vi "Process.vi"(9 "process sync":refnum<notifier>, 11 "Main in":refnum<class "Main.lvclass">) -> ()   [LabVIEW 2019, in "Main.lvclass"]
doc: "Developed by Kevin Thompson\nkevin@thompsonengineering.net\n\nCopyright 2018\nThompson Engineering, LLC"
uses:
  Main.lvclass
  <vilib>/TELLC/SMQ/Add States to Queue using MultiLine String with vData.vi
  DataTypes/Process - AppData--cluster.ctl
  Common/DataTypes/TD Async CmdMsg EventData--cluster.ctl
  DataTypes/Public Events--cluster.ctl
  DataTypes/Dependency--cluster.ctl
  DataTypes/Settings--cluster.ctl
  Log_Engine/Log_Engine.lvclass
  DAQ_Engine/DAQ_Engine.lvclass
  Config/Config.lvclass
  Common/DataTypes/RawChannelData--cluster.ctl
  Common/DataTypes/RawDAQData--cluster.ctl
  Common/DataTypes/ChannelWaveforms--cluster.ctl
  Common/DataTypes/InverterWaveforms--cluster.ctl
  Common/DataTypes/InverterWaveforms--QRef.ctl
  Common/DataTypes/RawDAQDataQRef--cluster.ctl
  support/Data Algorithms/subvis/DataTypes/averaging variables.ctl
  support/Data Algorithms/subvis/DataTypes/ESR alarm variables.ctl
  support/Data Algorithms/subvis/DataTypes/Processing loop variables--cluster.ctl
  DataTypes/PrivateAsynEv_Main--enum.ctl
  Common/DataTypes/Measurement Config--cluster.ctl
  Common/DataTypes/DAQState--enum.ctl
  Common/DataTypes/Acquisition Mode--cluster.ctl
  support/Data Algorithms/subvis/DataTypes/Gain control.ctl
  Common/DataTypes/TDMSState--enum.ctl
  Common/DataTypes/LogState--enum.ctl
  Common/DataTypes/UpdateControlValue EvData--cluster.ctl
  support/Data Algorithms/subvis/DataTypes/ESR scaling--cluster.ctl
  DataTypes/DataProcessAuxData--cluster.ctl
  Common/DataTypes/DataProcAuxDat--Qref.ctl
  DataTypes/ProcessingState--enum.ctl
  DataTypes/ProcessingStateChg EvData--cluster.ctl
  DataTypes/InverterInfo--cluster.ctl
  DataTypes/ProcessInitParams--cluster.ctl
  DataTypes/StartProcInitParams--cluster.ctl
  Common/DataTypes/inverter offset range--cluster.ctl
  Common/DataTypes/inverter gain range--cluster.ctl
  Common/DataTypes/inverter info v2--cluster.ctl
  Common/DataTypes/Inverter database record v2--cluster.ctl
panel:
  in  "Data Rate 9775(S/s)":dbl=3.0 format="%#.6p"
  out "DAQ data":T1
  out "RawDaqDataQ size":i32
  in  "reset averaging":bool
  in  "Dummy Vrms":dbl=120.0
  in  "UseDummyVrms":bool
  in  "ESR scaling":T3[](array[typedef])
  in  "Data Rate 9215 (S/s)":dbl=1200000.0 format="%#.6p"
  in  "Signal scaling":T4[](array[typedef])
  in  "Exit":bool
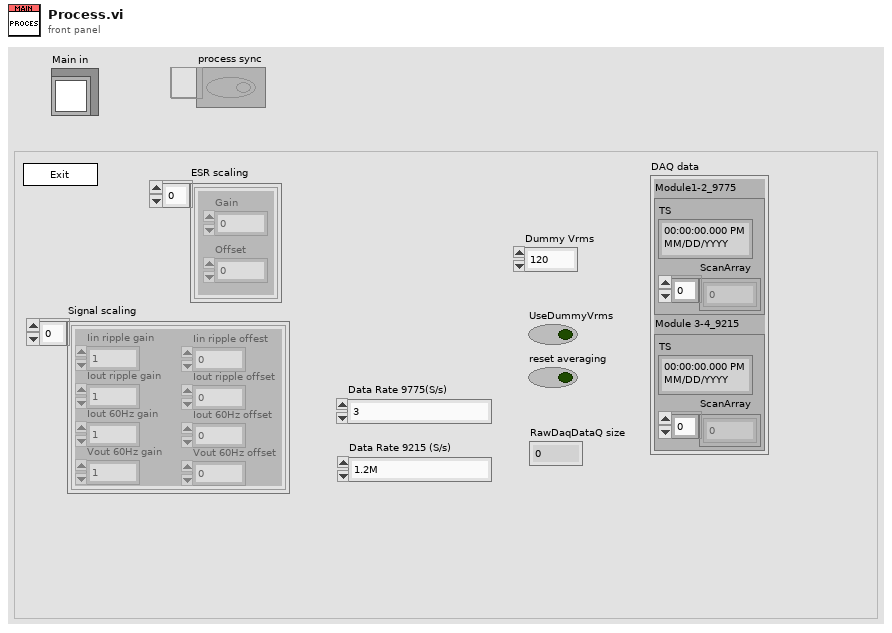
[diagram p1: front panel]
types:
  T1 = typedef "RawDAQData--cluster.ctl" = cluster{"Module1-2_9775":T2, "Module 3-4_9215":T2}
  T2 = typedef "RawChannelData--cluster.ctl" = cluster{"TS":timestamp, "ScanArray":dbl[]}
  T3 = typedef "Main.lvclass/ESR scaling--cluster.ctl" = cluster{"Gain":dbl, "Offset":dbl}
  T4 = typedef "Main.lvclass/Gain control.ctl" = cluster{"Iin ripple gain":dbl, "Iout ripple gain":dbl, "Iout 60Hz gain ":dbl, "Vout 60Hz gain ":dbl, "Iin ripple offest":dbl, "Iout ripple offset":dbl, "Iout 60Hz offset":dbl, "Vout 60Hz offset":dbl}
  T5 = typedef "Main.lvclass/ProcessingState--enum.ctl" = enum16{"Idle", "Starting", "Running", "Done", "Error"}
  T6 = typedef "Main.lvclass/Process - AppData--cluster.ctl" = cluster{"Core":cluster{"Current VI Reference":refnum<vi>, "Close Panel on Exit?":bool}, "Your Boolean data":bool, "Your string data":string, "SMQ":refnum<queue>, "Initialized?":bool, "Self Reference":refnum<class "Main.lvclass">, "Simulation?":bool, "process sync":refnum<notifier>, "vData":variant, "Settings":T7, "Dependency":T8, "Public Events":T9, "RawDaqDataQ":T10, "InverterWaveformsQ":T11, "Processing loop variables":T12, "Measurement config":T19, "Acquisition mode":T20, "DAQState":T21, "Signal scaling":T4, "PrivateAsync Ev":refnum<user-event>, "LogState":T22, "TDMSState":T23, "InvWfmsQ-DT":T11, "DPAuxDataQ":T24, "ProcessingState":T5, "InverterInfo":T25, "ProcLoopInterval":u32, "StoredESR Baseline":dbl[], "StoreESR BLine Flag":bool, "UseSavedESR BLine Flag":bool}
  T7 = typedef "Main.lvclass/Settings--cluster.ctl" = cluster{"Simulation":bool, "Signal scaling":T4[], "ESR scaling":T3[], "num readings to average":i32[], "ESR alarm threshhold (%)":i32[], "UseDummyVrms":bool, "Dummy Vrms":dbl, "Inverter Database File":path, "default Inverter (name)":string[], "Minimum Current Threshold ":dbl[], "Sensors Database File":path, "default Sensors (name)":string[]}
  T8 = typedef "Main.lvclass/Dependency--cluster.ctl" = cluster{"Config":refnum<class "Config.lvclass">, "DAQ":refnum<class "DAQ_Engine.lvclass">, "Log_Engine":refnum<class "Log_Engine.lvclass">}
  T9 = typedef "Main.lvclass/Public Events--cluster.ctl" = cluster{"Main.AsyncCmd Event":refnum<user-event>, "Main.AsyncMsg Event":refnum<user-event>, "stop process":refnum<user-event>, "UpdateControlValue Ev":refnum<user-event>, "ProcessingStateChg Ev":refnum<user-event>}
  T10 = typedef "RawDAQDataQRef--cluster.ctl" = refnum<queue>
  T11 = typedef "InverterWaveforms--QRef.ctl" = refnum<queue>
  T12 = typedef "Main.lvclass/Processing loop variables--cluster.ctl" = cluster{"DUT ESR avg":T13[], "DUT  PF avg":T13[], "DUT  Power avg ":T13[], "DUT processed data":cluster{"raw ESR":dbl, "Tcomp, avg ESR":dbl, "Vout RMS":dbl, "Iout RMS":dbl, "power factor":dbl, "power":dbl, "efficiency":dbl}[], "ESR alarm variables":T14[], "Status data":cluster{"Inv. 1 on?":bool, "Inv. 1 ESR over threshhold?":bool, "Minimum current":dbl}[], "CurrInverter":T15[], "miscellaneous":cluster{"Inverter 1 ID":string, "Inverter 2 ID":string, "Packet count":u32, "Calibration":dbl, "Calibration Gain":dbl, "Calibration Offset":dbl, "Calculated Total Power":dbl, "Seconds":dbl, "Last Tag Event":dbl, "Tag Event Time":dbl}[], "DUT INVERTER data":cluster{"Raw ESR sum":dbl, "scaled raw ESR sum":dbl, "scaled and averaged raw ESR sum":dbl, "Total power":dbl}[]}
  T13 = typedef "Main.lvclass/averaging variables.ctl" = cluster{"raw value buffer":dbl[], "buffer index":i32, "Avg value":dbl, "num to avg":i32}
  T14 = typedef "Main.lvclass/ESR alarm variables.ctl" = cluster{"Inv 1 baseline ESR":dbl, "Inv 1 over threshold?":bool, "Alarm on?":bool, "inv 1 esr chart range":dbl, "inv 1 esr saved baseline":dbl, "ESR alarm threshhold":dbl}
  T15 = typedef "Inverter database record v2--cluster.ctl" = cluster{"name":string, "last updated":timestamp, "type":string, "inverter Info":T16, "gain range":T17, "offset range":T18, "gain actual":dbl, "offset actual":dbl, "power level":dbl, "minimum current":dbl, "resistance single phase":dbl, "resistance 3 phase":dbl, "set flag":u16}
  T16 = typedef "inverter info v2--cluster.ctl" = cluster{"manufacturer":string, "model":string, "product":string, "serial":string, "power class":string, "year manf":string}
  T17 = typedef "inverter gain range--cluster.ctl" = cluster{"gain max":dbl, "gain min":dbl, "gain increment":dbl}
  T18 = typedef "inverter offset range--cluster.ctl" = cluster{"offset max":dbl, "offset min":dbl, "offset increment":dbl}
  T19 = typedef "Measurement Config--cluster.ctl" = cluster{"Data Rate 9775":dbl, "Data Rate 9215":dbl, "Samples RMS 9215":u32, "Samples RMS 9775":u32}
  T20 = typedef "Acquisition Mode--cluster.ctl" = enum16{"3phase", "Single"}
  T21 = typedef "DAQState--enum.ctl" = enum16{"Unknown", "Stopped", "Running", "Error"}
  T22 = typedef "LogState--enum.ctl" = enum16{"Unknown", "Stopped", "Running", "Error"}
  T23 = typedef "TDMSState--enum.ctl" = enum16{"Unknown", "Stopped", "Running", "Error"}
  T24 = typedef "DataProcAuxDat--Qref.ctl" = refnum<queue>
  T25 = typedef "InverterInfo--cluster.ctl" = cluster{"Inverter ID":string}
  T26 = typedef "Main.lvclass/ObjData--cluster.ctl" = cluster{"Settings":T7, "Public Events":T9, "Dependency":T8, "ReadData-placeholder":T27, "VISA-placeholder":refnum<visa-resource-name>, "InverterWaveformsQ":T11, "Application.TerminateProcess Event":refnum<user-event>, "RawDaqDataQ":T10, "MeasSettings":T19, "InverterDataAcqMode":T20, "DAQState Data":T28, "Private Events":T29, "InvWfmsQ-DT":T11, "DPAuxDataQ":T24, "ProcessingState":T5, "InverterInfo":T25, "CurrInverters":T15[], "InverterLUT Dict":T30, "ESR Chart Ref":refnum<vi>[], "StoreESR BLine Ref":refnum<vi>, "UseSavedESR BLine Ref":refnum<vi>, "CurrSensor":T31}
  T27 = typedef "Main.lvclass/Read Data--cluster.ctl" = cluster{"Data":dbl}
  T28 = typedef "DAQ_Engine.lvclass/DAQStateEvData--cluster.ctl" = cluster{"DAQState":T21, "vData":variant}
  T29 = typedef "Main.lvclass/Private Events--cluster.ctl" = cluster{"PrivateAsync Ev":refnum<user-event>}
  T30 = typedef "TD Dynamic CVT DVR--ref.ctl" = refnum<data-value>
  T31 = typedef "Sensor LUT--cluster.ctl" = cluster{"name":string, "last updated":timestamp, "manufacturer":string, "model":string, "Sensitivity index":dbl, "Sensor Ranges":T32}[]
  T32 = typedef "Sensor ranges--cluster.ctl" = cluster{"Max.VOut.RMS (V)":dbl, "Max.Out.Peak (V)":dbl, "Sensitivity (mV/A)":dbl, "Max.IOut.RMS(A)":dbl, "Min.IOut.RMS(A)":dbl}
  T33 = enum16{"Event Loop -", "Async Loop -", "DataProc Loop - "}
  T34 = typedef "Main.lvclass/PrivateAsynEv_Main--enum.ctl" = enum16{"PrivMain.UpdateMeasSettings", "PrivMain.UpdateAcqMode", "PrivMain.UpdateDAQState", "PrivMain.UpdateLogState", "PrivMain.UpdateTDMSState", "PrivMain.UpdateProcessingState", "PrivMain.Stop&Terminate", "PrivMain.CurrInverterUpdated", "PrivMain.UpdateStoreUseESRBaseline", "PrivMain.SetUnsetAlarm&ESRBLine", "PrivMain.ResetAveraging"}
  T35 = cluster{"VoltageDyn":dbl, "CurrentDyn":dbl, "MotorV SP":dbl}[]
  T36 = cluster{"Inv. 1 on?":bool, "Inv. 1 ESR over threshhold?":bool, "Minimum current":dbl}[]
  T37 = cluster{"Raw ESR sum":dbl, "scaled raw ESR sum":dbl, "scaled and averaged raw ESR sum":dbl, "Total power":dbl}[]
  T38 = typedef "InverterWaveforms--cluster.ctl" = T39[]
  T39 = typedef "ChannelWaveforms--cluster.ctl" = cluster{"Iin ripple ":waveform(dbl), "Iout ripple ":waveform(dbl), "Iout 60Hz":waveform(dbl), "Vout 60Hz":waveform(dbl)}
  T40 = typedef "DataProcessAuxData--cluster.ctl" = cluster{"Time Stamp":timestamp, "Raw ESR sum":dbl, "Inv 1 ON?":bool, "Average scaled ESR sum":dbl, "Inv 1 over threshold?":bool, "Inv 1 ESR":cluster{"ESR Baseline":dbl, "Alarm threshhold (%)":dbl, "Avg value":dbl}, "Max ESR":dbl}
  T41 = typedef "TD MeasData--cluster.ctl" = cluster{"Timestamp":timestamp, "ESR_Ohm":dbl[], "DUT data":T42[], "DUT INVERTER data":cluster{"Raw ESR sum":dbl, "scaled raw ESR sum":dbl, "scaled and averaged raw ESR sum":dbl, "Total power":dbl}[]}
  T42 = typedef "InverterPhaseData--cluster.ctl" = cluster{"RawESR_Ohm":dbl, "TcompAvgESR_Ohm":dbl, "VoutRMS_V":dbl, "IoutRMS_A":dbl, "PF":dbl, "AvgPF":dbl, "Power_W":dbl, "AvgPower_W":dbl, "efficiency":dbl}
  T43 = enum32{"invalid app kind", "Development System", "Run Time System", "Student Edition", "Embedded LabVIEW", "Evaluation", "Custom"}
  T44 = enum32{"Invalid", "Standard", "Closed", "Hidden", "Minimized", "Maximized"}
  T45 = cluster{"Inv. 1 on?":bool, "Inv. 1 ESR over threshhold?":bool, "Minimum current":dbl}
  T46 = cluster{"Inverter 1 ID":string, "Inverter 2 ID":string, "Packet count":u32, "Calibration":dbl, "Calibration Gain":dbl, "Calibration Offset":dbl, "Calculated Total Power":dbl, "Seconds":dbl, "Last Tag Event":dbl, "Tag Event Time":dbl}
  T47 = typedef "Main.lvclass/AsynCmd_Main--enum.ctl" = enum16{"Main.StartProcessing", "Main.StopProcessing", "Main.RefreshInverterList"}
  T48 = typedef "Main.lvclass/StartProcInitParams--cluster.ctl" = cluster{"InverterInfo":T25[], "ProcessInitParams":T49[]}
  T49 = typedef "Main.lvclass/ProcessInitParams--cluster.ctl" = cluster{"MinCurrThreshold":dbl, "NumPF RdsToAvg":i32, "ESR alarm threshhold (%)":dbl, "# readings to average":i32}
  T50 = typedef "Main.lvclass/AsynMsg_Main--enum.ctl" = enum16{"Main.CurrInverterUpdated"}
  T51 = typedef "DAQ_Engine.lvclass/DAQMeasSettingsEvData--cluster.ctl" = cluster{"Measurement config":T19, "vData":variant}
  T52 = typedef "Log_Engine.lvclass/LogStateEvData--cluster.ctl" = cluster{"LogState":T22, "vData":variant}
  T53 = typedef "Log_Engine.lvclass/TDMSStateEvData--cluster.ctl" = cluster{"TDMSState":T23, "vData":variant}
  T54 = typedef "DAQ_Engine.lvclass/Public Events--cluster.ctl" = cluster{"DAQ_Engine.AsyncCmd Event":refnum<user-event>, "DAQ_Engine.AsyncMsg Event":refnum<user-event>, "stop process":refnum<user-event>, "DAQ_Engine.DAQStateChg Ev":refnum<user-event>, "DAQ_Engine.MeasSettingsChg Ev":refnum<user-event>, "DAQ_Engine.AcqModeChg Ev":refnum<user-event>}
  T55 = typedef "Log_Engine.lvclass/Public Events--cluster.ctl" = cluster{"Log_Engine.AsyncCmd Event":refnum<user-event>, "Log_Engine.AsyncMsg Event":refnum<user-event>, "stop process":refnum<user-event>, "Log_Engine.LogStateChg Ev":refnum<user-event>, "Log_Engine.TDMSStateChg Ev":refnum<user-event>}
  T56 = cluster{"Current VI Reference":refnum<vi>, "Close Panel on Exit?":bool}
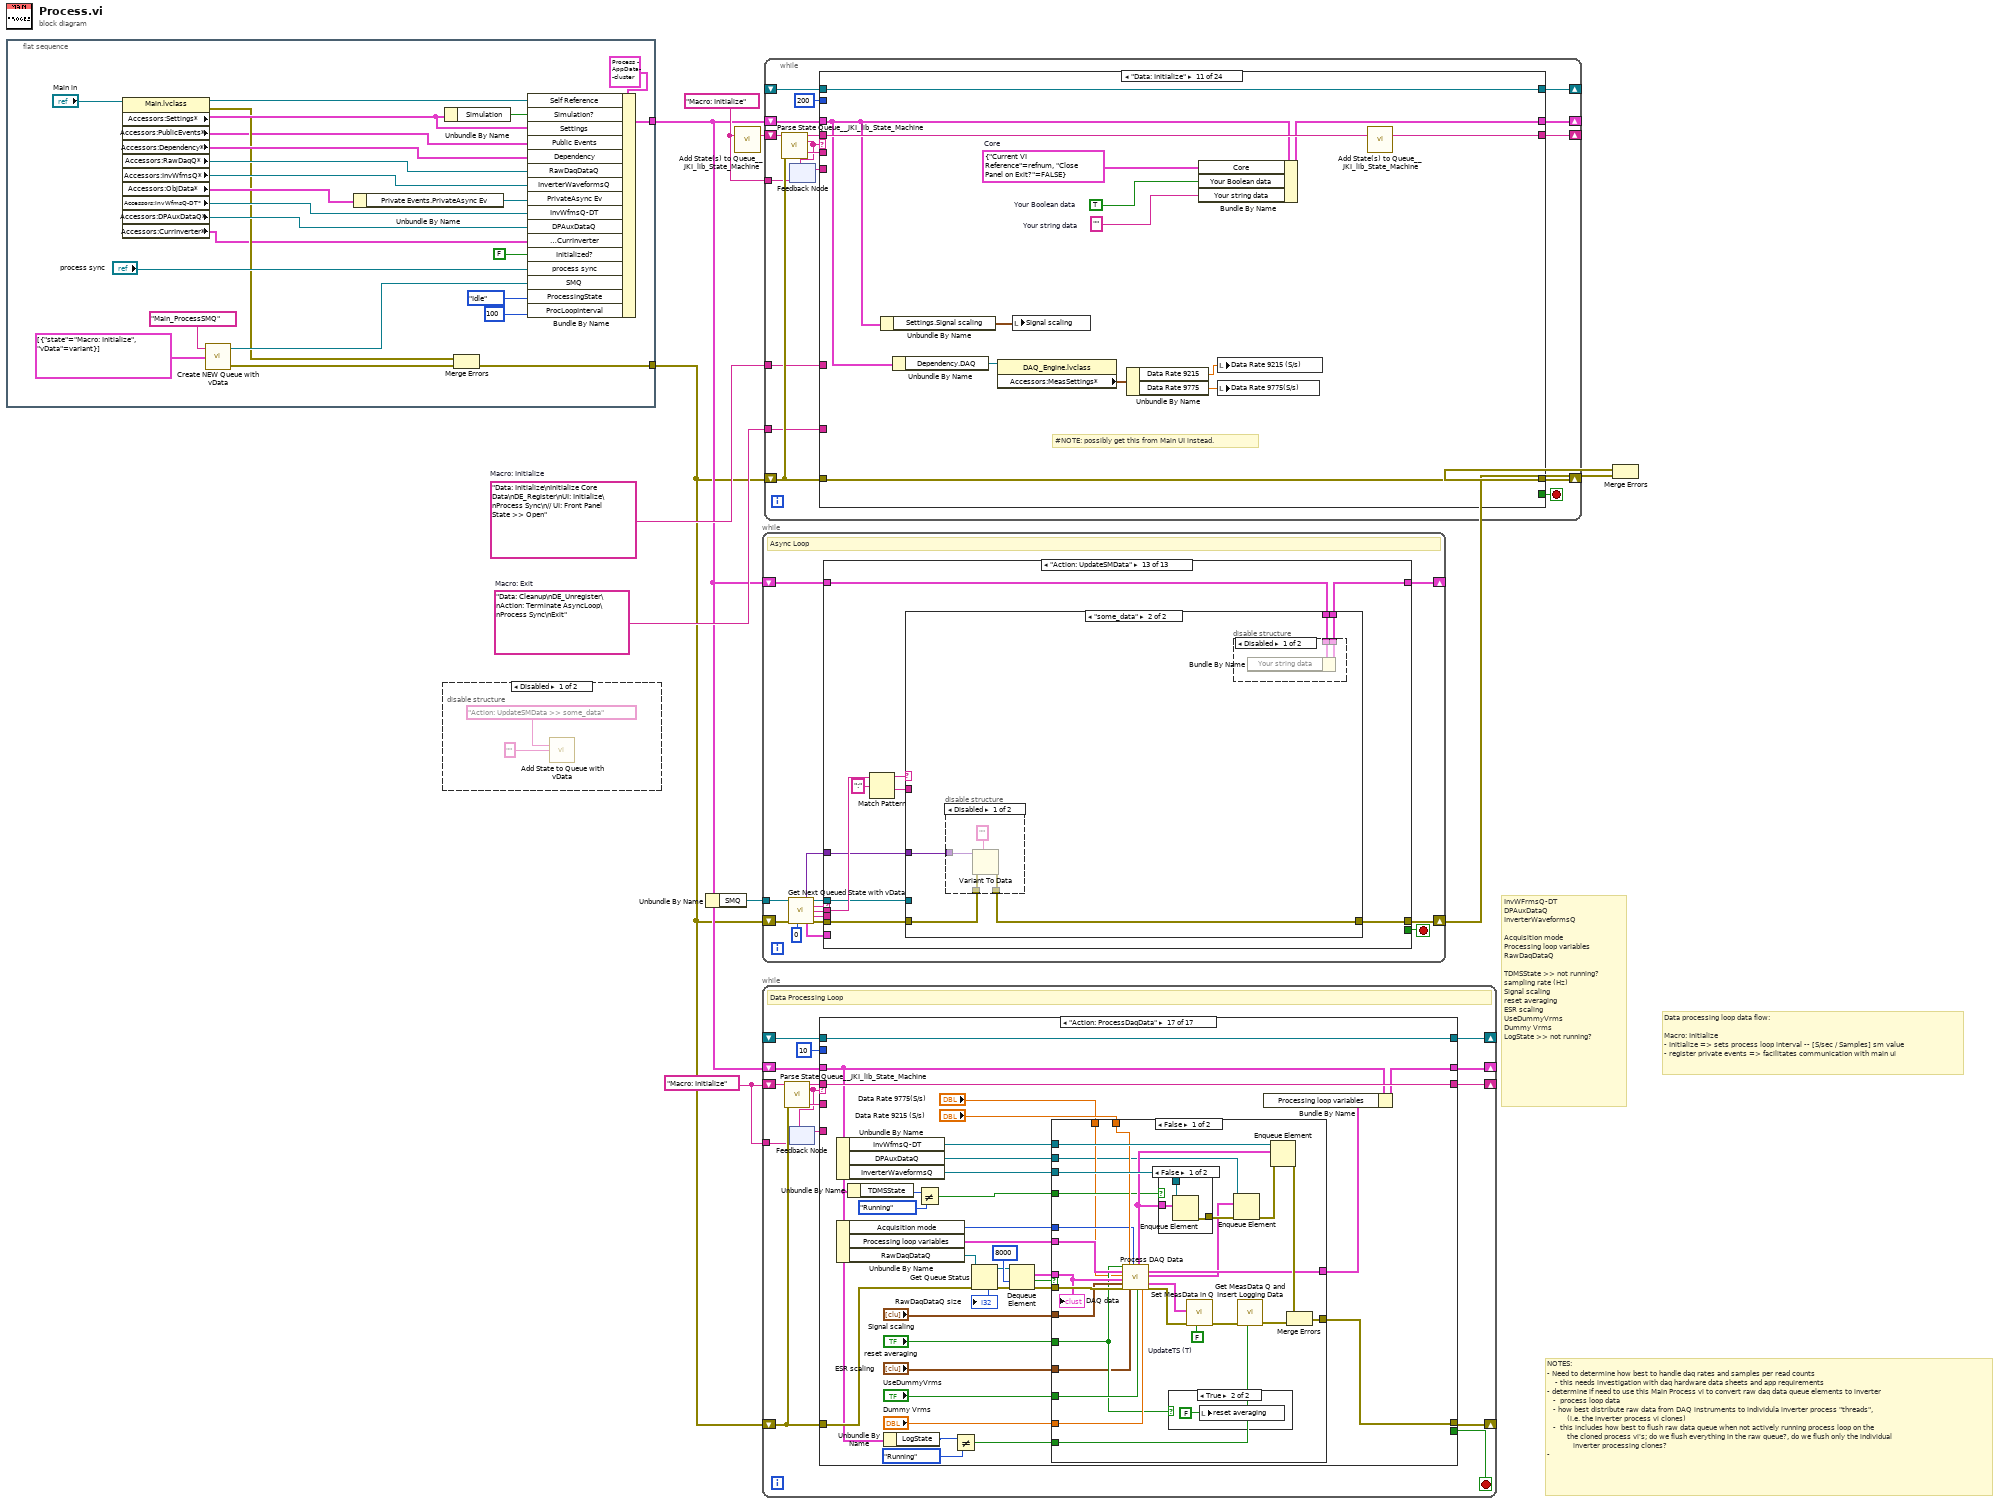
[diagram p0: block diagram]
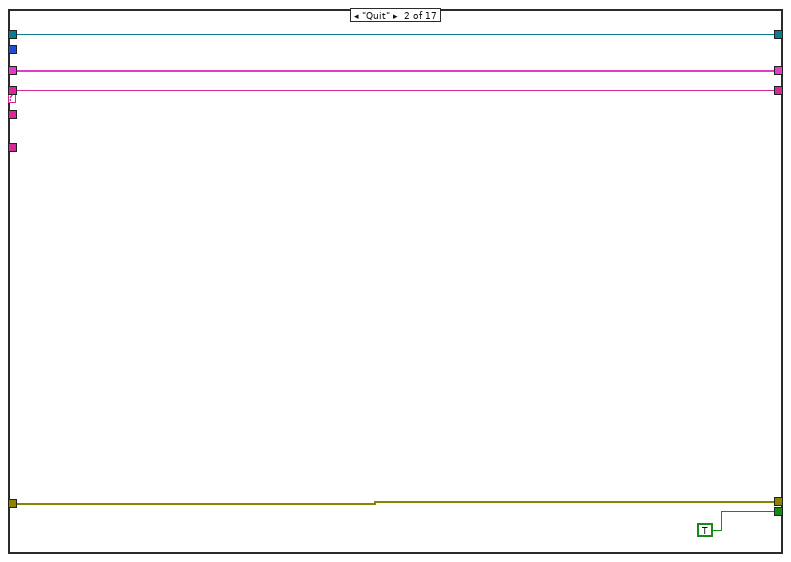
[diagram p3: hidden frame]
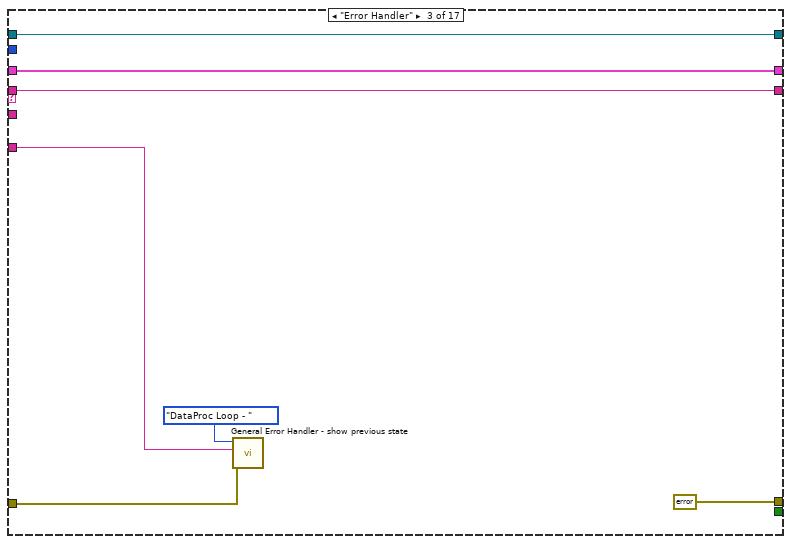
[diagram p4: hidden frame]
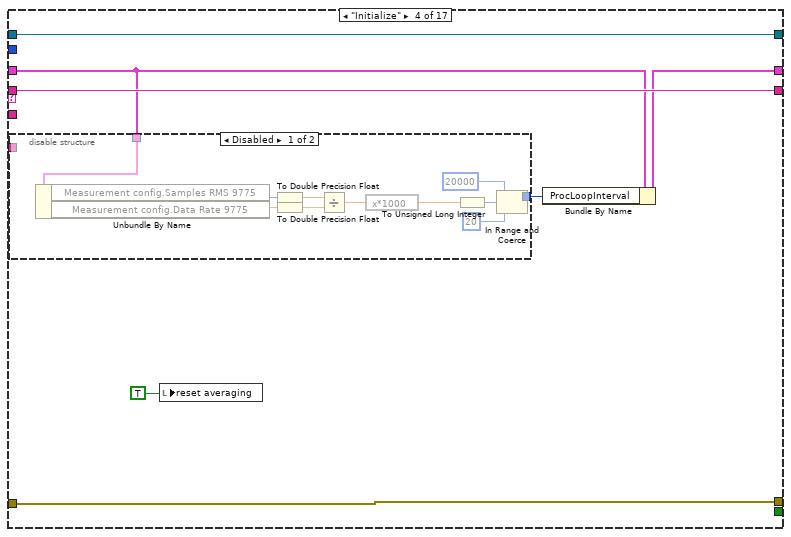
[diagram p5: hidden frame]
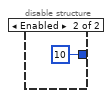
[diagram p6: hidden frame]
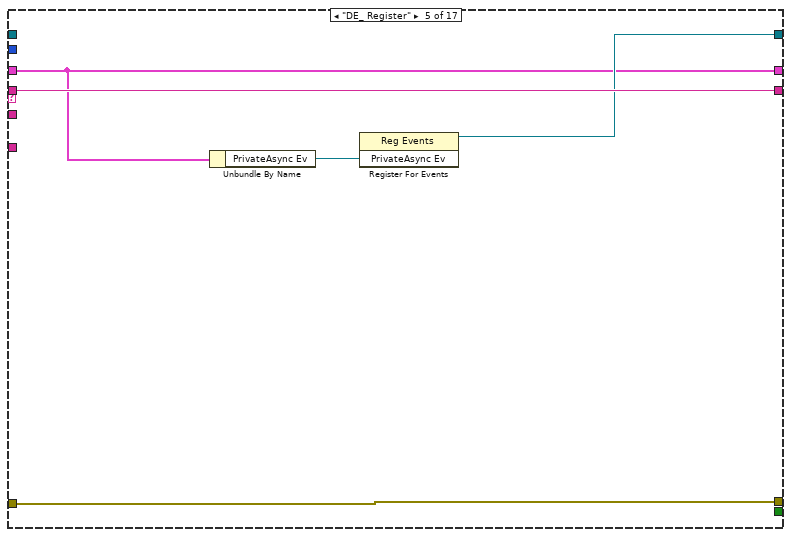
[diagram p7: hidden frame]
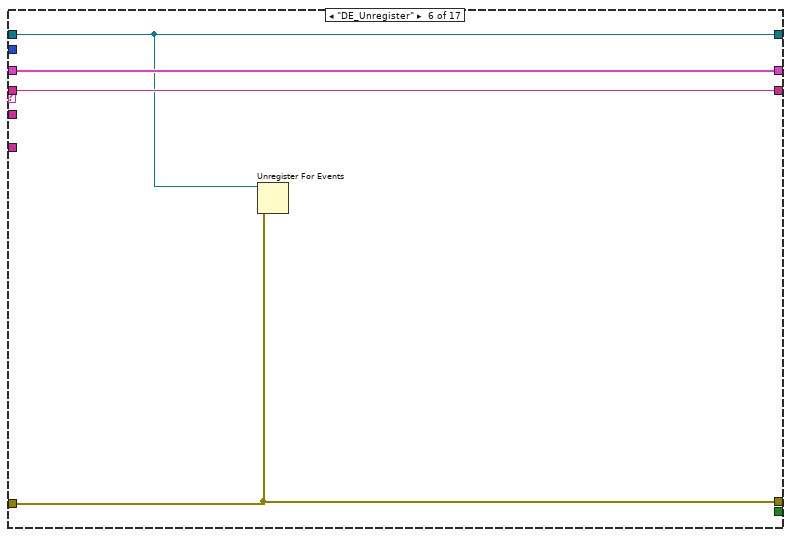
[diagram p8: hidden frame]
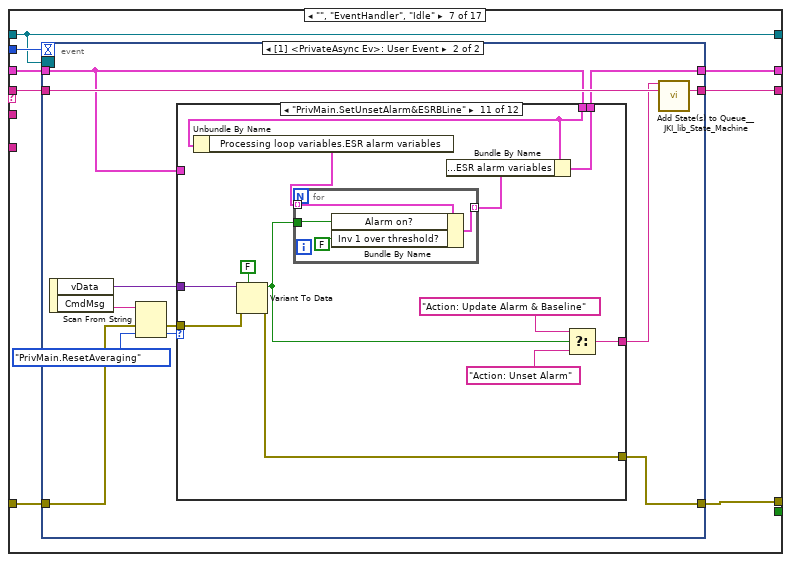
[diagram p9: hidden frame]
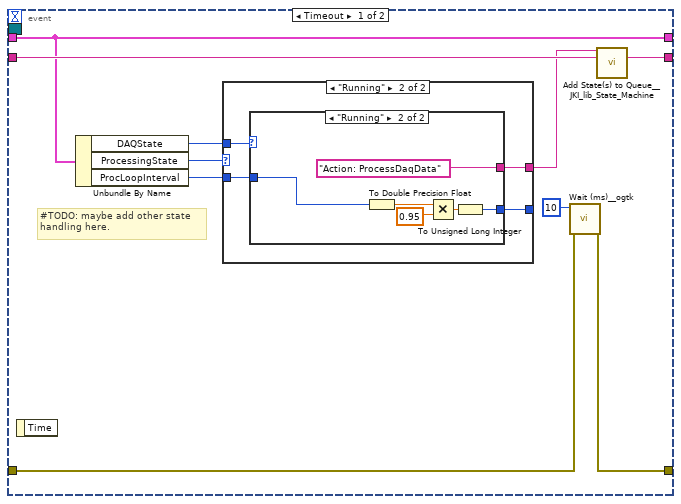
[diagram p10: hidden frame]
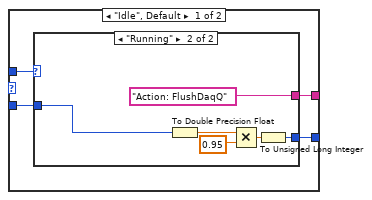
[diagram p11: hidden frame]
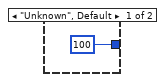
[diagram p12: hidden frame]
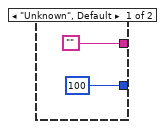
[diagram p13: hidden frame]
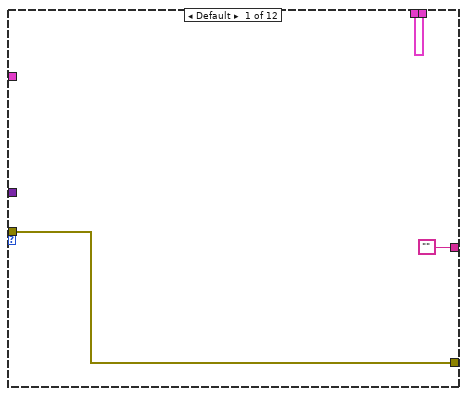
[diagram p14: hidden frame]
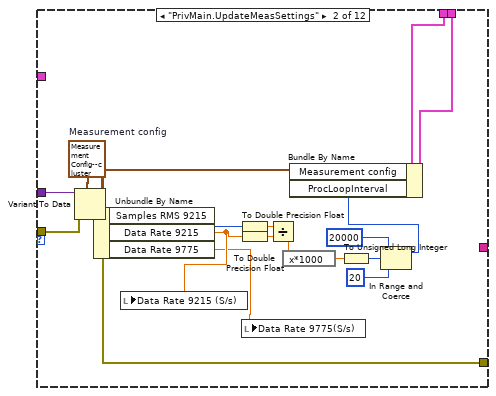
[diagram p15: hidden frame]
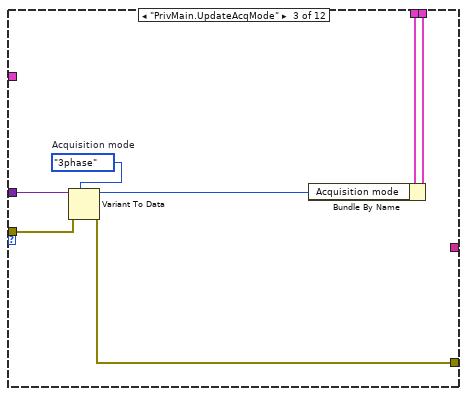
[diagram p16: hidden frame]
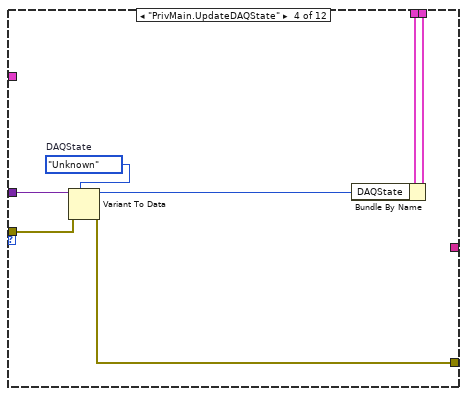
[diagram p17: hidden frame]
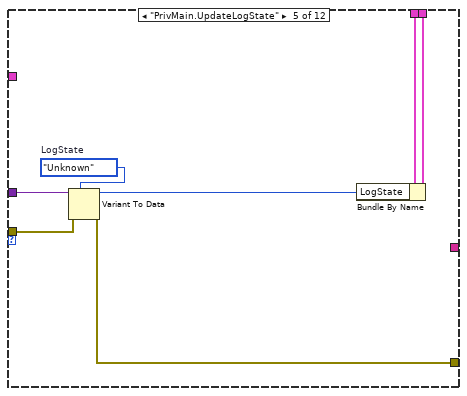
[diagram p18: hidden frame]
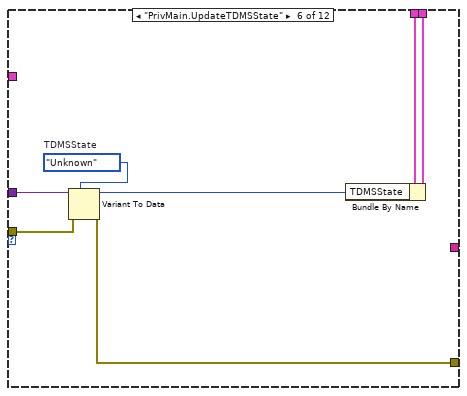
[diagram p19: hidden frame]
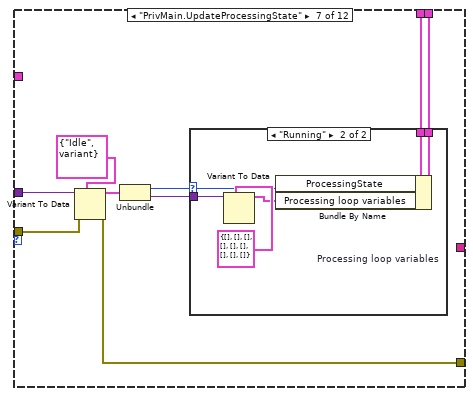
[diagram p20: hidden frame]
diagram:
  w1 = "Macro: Initialize"
  w8 = "Data: Cleanup\nDE_Unregister\nAction: Terminate AsyncLoop\nProcess Sync\nExit"  # Macro: Exit
  w9 = "Data: Initialize\nInitialize Core Data\nDE_Register\nUI: Initialize\nProcess Sync\n// UI: Front Panel State >> Open"  # Macro: Initialize
  w4 = "Macro: Initialize"
  # "NOTES:\n- Need to determine how best to handle daq rates and samples per read counts\n    - this needs investigation with daq hardware data sheets and app requirements\n- determine if need to use this Main Process vi to convert raw daq data queue elements to inverter\n   -  process loop data\n   - how best distribute raw data from DAQ instruments to individula inverter process \"threads\",\n          (i.e. the inverter process vi clones)\n   -  this includes how best to flush raw data queue when not actively running process loop on the\n          the cloned process vi's; do we flush everything in the raw queue?, do we flush only the individual\n             inverter processing clones?\n-"
  # "Data processing loop data flow:\n\nMacro: Initialize\n- Initialize => sets process loop interval -- [S/sec / Samples] sm value\n- register private events => facilitates communication with main ui"
  # "InvWFrmsQ-DT\nDPAuxDataQ\nInverterWaveformsQ\n\nAcquisition mode\nProcessing loop variables\nRawDaqDataQ\n\nTDMSState >> not running?\nsampling rate (Hz)\nSignal scaling\nreset averaging\nESR scaling\nUseDummyVrms\nDummy Vrms\nLogState >> not running?"
  n1 = flat-sequence {
    tunnel: [w35] -> w3
    tunnel: [w16] -> w2
    frame #0 {
      n2 = property class="Main.lvclass"(reference="Main in") -> (reference out=w14:refnum<class "Main.lvclass">, error out=w15:errorcluster, "Accessors:Settings*"=w26:T7, "Accessors:PublicEvents*"=w13:T9, "Accessors:Dependency*"=w28:T8, "Accessors:RawDaqQ*"=w24:T10, "Accessors:InvWfmsQ*"=w23:T11, "Accessors:ObjData*"=w22:T26, "Accessors:InvWfmsQ-DT*"=w20:T11, "Accessors:DPAuxDataQ*"=w19:T24, "Accessors:CurrInverter*"=w11:T15[])  [unwired: 1 in]
      n3 = call <vilib>:"Create NEW Queue with vData.vi"("Initial States"=cluster{"state":string, "vData":variant}[] [{"state"="Macro: Initialize", "vData"=variant}], "Name (SMQ)"="Main_ProcessSMQ") -> ("error out"=w32:errorcluster, "queue out"=w34:refnum<queue>)  [unwired: 2 in]
      n4 = Unbundle By Name(w22) -> ("Private Events.PrivateAsync Ev"=w21:refnum<user-event>)
      n5 = Unbundle By Name(w26) -> ("Simulation"=w27:bool)
      n6 = Merge Errors(w15, w32) -> (w16:errorcluster)
      n7 = Bundle By Name(cluster=T6 {"Core"={"Current VI Reference"=refnum, "Close Panel on Exit?"=FALSE}, "Your Boolean data"=FALSE, "Your string data"="", "SMQ"=refnum, "Initialized?"=FALSE, "Self Reference"=refnum, "Simulation?"=FALSE, "process sync"=refnum, "vData"=variant, "Settings"={"Simulation"=FALSE, "Signal scaling"=[], "ESR scaling"=[], "num readings to average"=[], "ESR alarm threshhold (%)"=[], "UseDummyVrms"=FALSE, "Dummy Vrms"=0.0, "Inverter Database File"=path "", "default Inverter (name)"=[], "Minimum Current Threshold "=[], "Sensors Database File"=path "", "default Sensors (name)"=[]}, "Dependency"={"Config"=refnum, "DAQ"=refnum, "Log_Engine"=refnum}, "Public Events"={"Main.AsyncCmd Event"=refnum, "Main.AsyncMsg Event"=refnum, "stop process"=refnum, "UpdateControlValue Ev"=refnum, "ProcessingStateChg Ev"=refnum}, "RawDaqDataQ"=refnum, "InverterWaveformsQ"=refnum, "Processing loop variables"={"DUT ESR avg"=[], "DUT  PF avg"=[], "DUT  Power avg "=[], "DUT processed data"=[], "ESR alarm variables"=[], "Status data"=[], "CurrInverter"=[], "miscellaneous"=[], "DUT INVERTER data"=[]}, "Measurement config"={"Data Rate 9775"=3.0, "Data Rate 9215"=1200000.0, "Samples RMS 9215"=480000, "Samples RMS 9775"=3}, "Acquisition mode"=enum."3phase", "DAQState"=enum."Unknown", "Signal scaling"={"Iin ripple gain"=13.333, "Iout ripple gain"=13.333, "Iout 60Hz gain "=14.286, "Vout 60Hz gain "=20.0, "Iin ripple offest"=0.0, "Iout ripple offset"=0.0, "Iout 60Hz offset"=0.0, "Vout 60Hz offset"=0.0}, "PrivateAsync Ev"=refnum, "LogState"=enum."Unknown", "TDMSState"=enum."Unknown", "InvWfmsQ-DT"=refnum, "DPAuxDataQ"=refnum, "ProcessingState"=enum."Idle", "InverterInfo"={"Inverter ID"=""}, "ProcLoopInterval"=0, "StoredESR Baseline"=[], "StoreESR BLine Flag"=FALSE, "UseSavedESR BLine Flag"=FALSE} ("SM2 AppData"), "Self Reference"=w14, "Simulation?"=w27, "Settings"=w26, "Public Events"=w13, "Dependency"=w28, "RawDaqDataQ"=w24, "InverterWaveformsQ"=w23, "PrivateAsync Ev"=w21, "InvWfmsQ-DT"=w20, "DPAuxDataQ"=w19, "Processing loop variables.CurrInverter"=w11, "Initialized?"=FALSE, "process sync"="process sync", "SMQ"=w34, "ProcessingState"=ProcessingState--enum."Idle", "ProcLoopInterval"=u32 100) -> (w35:T6)
    }
  }
  n8 = disable-structure shown="Disabled" {
    frame Disabled {
      n9 = call <vilib>:"Add State to Queue with vData.vi"("state in"="Action: UpdateSMData >> some_data", "vData (\"\")"="") -> ()  [unwired: 10 in, 4 out]
    }
    frame Enabled {
    }
  }
  n10 = Unbundle By Name(w3) -> ("SMQ"=w7:refnum<queue>)
  n11 = call <vilib>:"Add State(s) to Queue__JKI_lib_State_Machine.vi"("State(s) in (\"\")"=w4) -> ("States Out"=w10:string)  [unwired: 14 in]
  n12 = while {
    shift-right: [w48] -> w5
    shift-left: w2 -> [w50]
    tunnel: w7 -> [w46]
    shift-right: [w44] -> _
    shift-left: w3 -> [w45]
    stop <- w39 stop-if-true
    # "Async Loop"
    n13 = call <vilib>:"Get Next Queued State with vData.vi"("queue in"=w46, "error in (no error)"=w50, "timeout (100)"=0) -> ("vData out"=w43:variant, "queue out"=w47:refnum<queue>, "Next State"=w51:string, "queued msg"=w41:string, "Prev State"=w40:string, "RemainingElements"=w38:cluster{"state":string, "vData":variant}[], "error out"=w49:errorcluster)  [unwired: 6 in]
    n14 = case shown="\"Action: UpdateSMData\"" w51 {
      tunnel: w47 -> [_ _ _ _ w70 w80 _ w96 w101 _ _ _ w138]
      tunnel: w41 -> [_ _ _ _ _ _ _ _ _ _ _ w127 w140]
      selector: w51 -> [w52 _ _ _ _ _ _ _ _ _ _ _ _]
      tunnel: w49 -> [w54 w62 w64 w69 w76 w78 w92 w95 w100 w104 w106 w126 w135]
      tunnel: [w53 w62 errorcluster {"status"=FALSE, "code"=0, "source"=""} ("error constant") w69 w76 w77 w92 w94 w99 w104 w106 w129 w134] -> w48
      tunnel: w45 -> [w60 w61 w67 w68 w75 w79 w91 w97 w102 w103 w107 w132 w137]
      tunnel: [w60 w61 w67 w68 w75 w79 w91 w97 w102 w103 w107 w132 w136] -> w44
      tunnel: w43 -> [_ _ _ _ _ _ _ _ _ _ _ _ w139]
      tunnel: w40 -> [_ _ w63 _ _ _ _ _ _ _ _ _ _]
      tunnel: [_ _ _ _ TRUE _ _ _ _ _ _ _ _] -> w39
      tunnel: w38 -> [_ _ _ _ _ _ _ _ _ _ _ _ _]
      frame Default {
        w56 = 42 items=["No error", "Argument error", "Memory is full", "Out of zone", "End of file", "File already open", "Generic file I/O error", "File not found", "File permission error", "Disk is full", "Duplicate path", "Too many files open", "System feature not enabled", "Resource file not found", "Cannot add resource", "Resource not found", "Image not found", "Image memory error", "Pen does not exist", "Config type invalid", "Config token not found", "Config parse error", "Config memory error", "Bad external code format", "Bad external code offset", "External code not present", "Null window", "Destroy window error", "Null menu", "Print aborted", "Bad print record", "Print driver error", "Windows error during printing", "Memory error during printing", "Print dialog error", "Generic print error", "Invalid device refnum", "Device not found", "Device parameter error", "Device unit error", "Cannot open device", "Device call aborted", "Generic error", "Cancelled by user", "Object ID too low", "Object ID too high", "Object not in heap", "Unknown heap", "Unknown object (invalid DefProc)", "Unknown object (DefProc not in table)", "Message out of range", "Invalid (null) method", "Unknown message", "Manager call not supported", "Bad address", "Network operation in progress", "Network operation timed out", "Connection is busy", "Network attribute not supported", "Network error", "Address in use", "System out of memory", "Connection aborted", "Connection refused", "Not connected", "Already connected", "Connection closed", "Initialization error (interapplication manager)", "Bad occurrence", "Wait on unbound occurrence handler", "Occurrence queue overflow", "Datalog type conflict", "Unused", "Unrecognized type (interapplication manager)", "Memory corrupt", "Failed to make temporary DLL", "Old CIN version", "Drag socket not found", "Failed to load drop-object", "Failed to register OLE object", "Failed to release OLE object", "Format specifier type mismatch", "Unknown format specifier", "Too few format specifiers", "Too many format specifiers", "Scan failed", "Newer CIN version", "Error converting to variant", "Runtime menu error", "Password tampered", "Variant attribute not found", "Incompatible variant data type", "Event data is not available", "Event Store is not present", "Occurrence is not found", "Event Queue is not created", "Event info is not available", "Refnum passed is NULL", "Error retrieving Class GUID", "Error retrieving CoClass GUID", "Error retrieving TypeLib GUID.", "Bad built application magic bytes.", "Specific driver is different from the specific driver associated with the Logical Name.", "There is no session opened to the class driver.", "Max Error", "MAX - Error with config objects", "MAX - Error loading configuration", "MAX - Group not supported"]
        n15 = Format Into String(format string="Software Exception: Unhandled State \"%s\"." ("message"), error in=w54, w52) -> (resulting string=w57:string, error out=w58:errorcluster)  [unwired: 1 in]
        n16 = call <vilib>:"Error Cluster From Error Code.vi"("show call chain? (False)"=TRUE, "error in (no error)"=w58, "error message (\"\")"=w57, "error code (0)"=w56) -> ("error out"=w53:errorcluster)  [unwired: 5 in]
      }
      frame "Initialize" {
      }
      frame "Error Handler" {
        n17 = call "General Error Handler - show previous state.vi"("error in (no error)"=w64, "Previous State"=w63, "Loop Select"=enum16{"Event Loop -", "Async Loop -"}."Async Loop -") -> ()  [unwired: 7 in, 2 out]
      }
      frame "CleanUp" {
      }
      frame "Exit" {
        n18 = Flush Queue(queue=w70) -> (queue out=w73:refnum<queue>, error out=w72:errorcluster)  [unwired: 1 in, 1 out]
        n19 = Release Queue(queue=w73, force destroy? (F)=TRUE, error in (no error)=w72) -> ()  [unwired: 3 out]
      }
      frame "", "Idle" {
        # "#NOTE: This Async Loop NOT USED in this app.\nNeeded faster response; see bottom loop.\nCode remains here for reference and re-use if needed."
        # "#TODO: add condition"
        n20 = Unbundle By Name(w79) -> ()  [unwired: 1 out]
        n21 = case shown="False" FALSE {
          tunnel: w80 -> [_ w90]
          tunnel: w78 -> [w83 w87]
          tunnel: [w82 w85] -> w77
          frame False {
            n22 = call <userlib>:"Wait (ms)__ogtk.vi"("error in (no error)"=w83, "milliseconds to wait"=u32 200) -> ("error out"=w82:errorcluster)  [unwired: 8 in, 1 out]
          }
          frame True {
            n23 = call <userlib>:"Wait (ms)__ogtk.vi"("error in (no error)"=w87, "milliseconds to wait"=u32 50) -> ("error out"=w88:errorcluster)  [unwired: 8 in, 1 out]
            n24 = call-poly <vilib>:"Polymorphic - Add States(s) To Queue.vi"("queue in"=w90, "state in"="Action: ReadRawDaqQueue", "error in"=w88) -> ("error out"=w85:errorcluster)  [unwired: 9 in, 3 out]
          }
        }
      }
      frame "------ Macro ------" {
      }
      frame "Macro: Initialize" {
        n25 = call-poly <vilib>:"Polymorphic - Add States(s) To Queue.vi"("queue in"=w96, "states in"="Initialize\n/* some state\n/* another state\nIdle", "error in"=w95) -> ("error out"=w94:errorcluster)  [unwired: 10 in, 2 out]
      }
      frame "Macro: Exit" {
        n26 = call-poly <vilib>:"Polymorphic - Add States(s) To Queue.vi"("queue in"=w101, "states in"="/* some state\n/* another state\nCleanUp\nExit", "error in"=w100) -> ("error out"=w99:errorcluster)  [unwired: 10 in, 2 out]
      }
      frame "------ Action ------" {
      }
      frame "Action: ReadRawDaqQueue" {
        n27 = Unbundle By Name(w107) -> ("RawDaqDataQ"=w105:T10)
        n28 = disable-structure shown="Disabled" {
          disable-tunnel: w105 -> [_ w108 w119]
          frame Enabled {
          }
          frame Disabled {
            n29 = Get Queue Status(queue=w108) -> (queue out=w110:T10, error out=w109:errorcluster, # elements in queue=w111:i32)  [unwired: 2 in, 5 out]
            n30 = case shown="1, Default" w111 {
              selector: w111 -> [_ w114]
              tunnel: w110 -> [_ w113]
              tunnel: w109 -> [_ w112]
              frame 0 {
              }
              frame 1, Default {
                n31 = for {
                  N: w114 -> [_]
                  tunnel: w113 -> [w118]
                  shift-right: [w116] -> _
                  shift-left: w112 -> [w117]
                  tunnel: [w115] -> _ mode=indexing
                  n32 = Dequeue Element(queue=w118, error in (no error)=w117) -> (element=w115:T1, error out=w116:errorcluster)  [unwired: 1 in, 2 out]
                }
              }
            }
          }
          frame Disabled {
            n33 = while {
              tunnel: w119 -> [w124]
              stop <- w123 stop-if-true
              n34 = Dequeue Element(queue=w124, timeout in ms (-1)=5) -> (timed out?=w122:bool, error out=w121:errorcluster)  [unwired: 1 in, 2 out]
              n35 = Compound Arithmetic op=OR(w122, w121) -> (w123:bool)
            }
          }
        }
      }
      frame "Action: Wait" {
        n36 = Scan From String(format string="%d", input string=w127, error in=w126, default 1=u32 0) -> (error out=w125:errorcluster, output 1=w131:u32)  [unwired: 1 in, 2 out]
        n37 = call <userlib>:"Wait (ms)__ogtk.vi"("error in (no error)"=w125, "milliseconds to wait"=w131) -> ("error out"=w129:errorcluster)  [unwired: 8 in, 1 out]
      }
      frame "Action: UpdateSMData" {
        n38 = Match Pattern(string=w140, regular expression=":") -> (before substring=w142:string, after substring=w133:string)  [unwired: 1 in, 2 out]
        n39 = case shown="\"some_data\"" w142 {
          tunnel: w139 -> [_ w149]
          tunnel: w138 -> [_ _]
          tunnel: w137 -> [w143 w148]
          tunnel: [w143 w147] -> w136
          tunnel: w135 -> [w144 w146]
          tunnel: [w144 w145] -> w134
          tunnel: w133 -> [_ _]
          frame Default {
            # "#NOTE:\noptionally add error here."
          }
          frame "some_data" {
            n40 = disable-structure shown="Disabled" {
              disable-tunnel: w149 -> [w156 _]
              disable-tunnel: w146 -> [w154 w157]
              disable-tunnel: [w153 w157] -> w145
              frame Disabled {
                n41 = Variant To Data(error in=w154, type="", Variant=w156) -> (error out=w153:errorcluster)  [unwired: 1 out]
              }
              frame Enabled {
              }
            }
            n42 = disable-structure shown="Disabled" {
              disable-tunnel: w148 -> [w151 w152]
              disable-tunnel: [w150 w152] -> w147
              frame Disabled {
                n43 = Bundle By Name(cluster=w151) -> (w150:T6)  [unwired: 1 in]
              }
              frame Enabled {
              }
            }
          }
        }
      }
    }
  }
  n44 = while {
    shift-right: [w171] -> _
    shift-left: w3 -> [w172]
    shift-right: [w170] -> _
    shift-left: w2 -> [w167]
    shift-right: [w165] -> _
    shift-left: w1 -> [w169]
    shift-right: [w163] -> _
    shift-left: _ -> [w162]
    tunnel: w1 -> [w158]
    stop <- w164 stop-if-true
    # "Data Processing Loop"
    n45 = call <vilib>:"Parse State Queue__JKI_lib_State_Machine.vi"("State Queue"=w169, "Error In (no error)"=w167) -> ("Remaining States"=w166:string, "Current State"=w160:string, "Arguments"=w168:string)  [unwired: 11 in]
    n46 = feedback #1(w158) -> (w159:string)
    n47 = feedback-in #1(w160) -> ()
    n48 = case shown="\"Action: ProcessDaqData\"" w160 {
      tunnel: w172 -> [w176 w181 w188 w190 w208 w216 w224 w385 w391 w397 w402 w406 w461 w486 w498 w518 w532]
      tunnel: [w176 w181 w188 w191 w208 w216 w223 w385 w391 w397 w402 w405 w461 w487 w497 w518 w537] -> w171
      tunnel: w167 -> [w175 w180 w184 w195 w212 w213 w222 w384 w390 w396 w401 w403 w454 w481 w501 w523 w538]
      tunnel: [w175 w180 errorcluster {"status"=FALSE, "code"=0, "source"=""} ("error constant") w195 w212 w213 w221 w384 w390 w396 w401 w404 w454 w482 w494 w523 w546] -> w170
      tunnel: w168 -> [_ _ _ _ _ _ _ _ _ _ _ _ _ _ _ w519 _]
      tunnel: w166 -> [w174 w179 w187 w193 w211 w215 w220 w383 w387 w393 w398 w407 w469 w492 w503 w522 w560]
      tunnel: [w174 w179 w187 w193 w211 w215 w219 w383 w388 w394 w399 w408 w470 w492 w504 w522 w560] -> w165
      tunnel: [_ TRUE _ _ _ _ _ _ _ _ _ _ _ _ _ _ _] -> w164
      tunnel: [w173 w177 w186 w194 w209 w214 w217 w382 w389 w395 w400 w409 w471 w491 w505 w521 w559] -> w163
      tunnel: w162 -> [w173 w177 w186 w194 _ w214 w217 w382 w389 w395 w400 w409 w471 w491 w505 w521 w559]
      tunnel: 10 -> [_ _ _ _ _ _ w218 _ _ _ _ _ _ _ _ _ _]
      tunnel: w159 -> [_ _ w183 _ _ _ _ _ _ _ _ _ _ _ _ _ _]
      frame Default {
      }
      frame "Quit" {
      }
      frame "Error Handler" {
        n49 = call "General Error Handler - show previous state.vi"("error in (no error)"=w184, "Previous State"=w183, "Loop Select"=T33."DataProc Loop - ") -> ()  [unwired: 7 in, 2 out]
      }
      frame "Initialize" {
        n50 = disable-structure shown="Disabled" {
          disable-tunnel: [w198 u32 10 ("upper limit")] -> w192
          disable-tunnel: w190 -> [w196 _]
          frame Disabled {
            n51 = Unbundle By Name(w196) -> ("Measurement config.Samples RMS 9775"=w206:u32, "Measurement config.Data Rate 9775"=w205:dbl)
            n52 = To Double Precision Float(number=w206) -> (double precision float=w203:dbl)
            n53 = To Double Precision Float(number=w205) -> (double precision float=w204:dbl)
            n54 = Divide(x=w203, y=w204) -> (x/y=w202:dbl)
            n55 = expression code="x*1000"(w202) -> (w201:dbl)
            n56 = To Unsigned Long Integer(number=w201) -> (unsigned 32bit integer=w200:u32)
            n57 = In Range and Coerce(upper limit=u32 20000, x=w200, lower limit=u32 20) -> (coerced(x)=w198:u32)  [unwired: 1 out]
          }
          frame Enabled {
          }
        }
        n58 = local write "reset averaging"(TRUE) -> ()
        n59 = Bundle By Name(cluster=w190, "ProcLoopInterval"=w192) -> (w191:T6)
      }
      frame "DE_ Register" {
        n60 = Unbundle By Name(w208) -> ("PrivateAsync Ev"=w210:refnum<user-event>)
        n61 = register-events(w210) -> (reference out=w209:refnum<event-registration>)  [unwired: 2 in, 1 out]
      }
      frame "DE_Unregister" {
        n62 = Unregister For Events(event registration refnum=w214, error in=w213) -> ()  [unwired: 1 out]
      }
      frame "", "EventHandler", "Idle" {
        n63 = event shown="[1] <PrivateAsync Ev>: User Event" {
          selector: w217 -> [_ _]
          dyn-events: _ -> [_ _]
          timeout: w218 -> [_ _]
          tunnel: w224 -> [w227 w258]
          tunnel: [w227 w262] -> w223
          tunnel: w222 -> [w228 w260]
          tunnel: [w229 w261] -> w221
          tunnel: w220 -> [w233 w264]
          tunnel: [w234 w263] -> w219
          event Timeout {
            # "#TODO: maybe add other state\nhandling here."
            n64 = event-data() -> ()  [unwired: 1 in, 1 out]
            n65 = Unbundle By Name(w227) -> ("DAQState"=w231:T21, "ProcessingState"=w230:T5, "ProcLoopInterval"=w226:u32)
            n66 = case shown="\"Running\"" w230 {
              tunnel: [w237 w249] -> w232
              tunnel: w231 -> [w238 w248]
              tunnel: w226 -> [w236 w247]
              tunnel: [w235 w246] -> _
              frame "Idle", Default {
                n67 = case shown="\"Running\"" w238 {
                  tunnel: [_ "Action: FlushDaqQ"] -> w237
                  tunnel: w236 -> [_ w243]
                  tunnel: [u32 100 w240] -> w235
                  frame "Unknown", Default {
                  }
                  frame "Running" {
                    n68 = To Double Precision Float(number=w243) -> (double precision float=w241:dbl)
                    n69 = Multiply(x=w241, y=0.95) -> (x*y=w244:dbl)
                    n70 = To Unsigned Long Integer(number=w244) -> (unsigned 32bit integer=w240:u32)
                  }
                }
              }
              frame "Running" {
                n71 = case shown="\"Running\"" w248 {
                  tunnel: ["" "Action: ProcessDaqData"] -> w249
                  tunnel: w247 -> [_ w253]
                  tunnel: [u32 100 ("ProcLoopInterval") w252] -> w246
                  frame "Unknown", Default {
                  }
                  frame "Running" {
                    n72 = To Double Precision Float(number=w253) -> (double precision float=w254:dbl)
                    n73 = Multiply(x=w254, y=0.95) -> (x*y=w256:dbl)
                    n74 = To Unsigned Long Integer(number=w256) -> (unsigned 32bit integer=w252:u32)
                  }
                }
              }
            }
            n75 = call <userlib>:"Wait (ms)__ogtk.vi"("error in (no error)"=w228, "milliseconds to wait"=u32 10) -> ("error out"=w229:errorcluster)  [unwired: 8 in, 1 out]
            n76 = call <vilib>:"Add State(s) to Queue__JKI_lib_State_Machine.vi"("State(s) in Front (\"\")"=w232, "State(s) in (\"\")"=w233) -> ("States Out"=w234:string)  [unwired: 13 in]
          }
          event User Event {
            n77 = event-data() -> ("vData"=w265:variant, "CmdMsg"=w269:string)  [unwired: 1 in]
            n78 = Scan From String(input string=w269, error in=w260, default 1=PrivateAsynEv_Main--enum."PrivMain.ResetAveraging" ("PrivAsync")) -> (error out=w266:errorcluster, output 1=w267:T34)  [unwired: 2 in, 2 out]
            n79 = case shown="\"PrivMain.SetUnsetAlarm&ESRBLine\"" w267 {
              tunnel: w266 -> [w270 w289 w296 w303 w310 w317 w326 w339 w345 w352 w367 w376]
              tunnel: w265 -> [_ w290 w297 w304 w311 w318 w327 _ w346 _ w368 w377]
              tunnel: w258 -> [w272 w287 w295 w302 w309 w316 w325 w338 w343 w353 w357 w374]
              tunnel: [w272 w286 w294 w301 w308 w315 w324 w338 w342 w351 w358 w374] -> w262
              tunnel: [w270 w285 w292 w299 w306 w313 w323 w339 w344 w348 w366 w375] -> w261
              tunnel: ["" _ _ _ _ _ _ "Macro: Exit" _ _ w363 _] -> w259
              tunnel: w258 -> [_ _ _ _ _ _ _ _ _ w347 _ _]
              frame Default {
              }
              frame "PrivMain.UpdateMeasSettings" {
                w288 = T19 {"Data Rate 9775"=3.0, "Data Rate 9215"=1200000.0, "Samples RMS 9215"=480000, "Samples RMS 9775"=3}  # Measurement config
                n80 = Variant To Data(error in=w289, type=w288, Variant=w290) -> (data=w284:T19, error out=w285:errorcluster)
                n81 = Unbundle By Name(w284) -> ("Samples RMS 9215"=w283:u32, "Data Rate 9215"=w274:dbl, "Data Rate 9775"=w273:dbl)
                n82 = local write "Data Rate 9215 (S/s)"(w274) -> ()
                n83 = To Double Precision Float(number=w283) -> (double precision float=w281:dbl)
                n84 = To Double Precision Float(number=w274) -> (double precision float=w282:dbl)
                n85 = local write "Data Rate 9775(S/s)"(w273) -> ()
                n86 = Divide(x=w281, y=w282) -> (x/y=w280:dbl)
                n87 = expression code="x*1000"(w280) -> (w279:dbl)
                n88 = To Unsigned Long Integer(number=w279) -> (unsigned 32bit integer=w278:u32)
                n89 = In Range and Coerce(upper limit=u32 20000, x=w278, lower limit=u32 20) -> (coerced(x)=w276:u32)  [unwired: 1 out]
                n90 = Bundle By Name(cluster=w287, "Measurement config"=w284, "ProcLoopInterval"=w276) -> (w286:T6)
              }
              frame "PrivMain.UpdateAcqMode" {
                w291 = Acquisition_Mode--cluster."3phase"  # Acquisition mode
                n91 = Variant To Data(error in=w296, type=w291, Variant=w297) -> (data=w293:T20, error out=w292:errorcluster)
                n92 = Bundle By Name(cluster=w295, "Acquisition mode"=w293) -> (w294:T6)
              }
              frame "PrivMain.UpdateDAQState" {
                w298 = DAQState--enum."Unknown"  # DAQState
                n93 = Variant To Data(error in=w303, type=w298, Variant=w304) -> (data=w300:T21, error out=w299:errorcluster)
                n94 = Bundle By Name(cluster=w302, "DAQState"=w300) -> (w301:T6)
              }
              frame "PrivMain.UpdateLogState" {
                w305 = LogState--enum."Unknown"  # LogState
                n95 = Variant To Data(error in=w310, type=w305, Variant=w311) -> (data=w307:T22, error out=w306:errorcluster)
                n96 = Bundle By Name(cluster=w309, "LogState"=w307) -> (w308:T6)
              }
              frame "PrivMain.UpdateTDMSState" {
                w312 = TDMSState--enum."Unknown"  # TDMSState
                n97 = Variant To Data(error in=w317, type=w312, Variant=w318) -> (data=w314:T23, error out=w313:errorcluster)
                n98 = Bundle By Name(cluster=w316, "TDMSState"=w314) -> (w315:T6)
              }
              frame "PrivMain.UpdateProcessingState" {
                n99 = Variant To Data(error in=w326, type=cluster{"ProcessingState":T5, variant} {"ProcessingState"=enum."Idle", variant}, Variant=w327) -> (data=w321:cluster{"ProcessingState":T5, variant}, error out=w323:errorcluster)
                n100 = Unbundle(w321) -> ("ProcessingState"=w319:T5, w320:variant)
                n101 = case shown="\"Running\"" w319 {
                  selector: w319 -> [w329 w331]
                  tunnel: w325 -> [w330 w336]
                  tunnel: [w328 w335] -> w324
                  tunnel: w320 -> [_ w334]
                  frame "Idle", Default {
                    # "Update ONLY the state which\nwill disable processing; leave\nthe loop var data alone."
                    n102 = Bundle By Name(cluster=w330, "ProcessingState"=w329) -> (w328:T6)
                  }
                  frame "Running" {
                    w333 = T12 {"DUT ESR avg"=[], "DUT  PF avg"=[], "DUT  Power avg "=[], "DUT processed data"=[], "ESR alarm variables"=[], "Status data"=[], "CurrInverter"=[], "miscellaneous"=[], "DUT INVERTER data"=[]}  # Processing loop variables
                    n103 = Variant To Data(type=w333, Variant=w334) -> (data=w332:T12)  [unwired: 1 in, 1 out]
                    n104 = Bundle By Name(cluster=w336, "ProcessingState"=w331, "Processing loop variables"=w332) -> (w335:T6)
                  }
                }
              }
              frame "PrivMain.Stop&Terminate" {
              }
              frame "PrivMain.CurrInverterUpdated" {
                n105 = Variant To Data(error in=w345, type=T15[] [], Variant=w346) -> (data=w341:T15[], error out=w344:errorcluster)
                n106 = Bundle By Name(cluster=w343, "Processing loop variables.CurrInverter"=w341) -> (w342:T6)
              }
              frame "PrivMain.UpdateStoreUseESRBaseline" {
                n107 = Unbundle By Name(w347) -> ("Self Reference"=w356:refnum<class "Main.lvclass">)
                n108 = call "Get StoreESR and UseSavedESR Flag reference.vi"("error in (no error)"=w352, "Main in"=w356) -> ("error out"=w348:errorcluster, "UseSavedESR BLine Ref"=w354:refnum<vi>, "StoreESR BLine Ref"=w355:refnum<vi>)  [unwired: 6 in, 1 out]
                n109 = property class="Bool (strict)"(reference=w355) -> ("Visible"=w350:bool)  [unwired: 1 in, 2 out]
                n110 = property class="Bool (strict)"(reference=w354) -> ("Visible"=w349:bool)  [unwired: 1 in, 2 out]
                n111 = Bundle By Name(cluster=w353, "StoreESR BLine Flag"=w350, "UseSavedESR BLine Flag"=w349) -> (w351:T6)
              }
              frame "PrivMain.SetUnsetAlarm&ESRBLine" {
                n112 = Unbundle By Name(w357) -> ("Processing loop variables.ESR alarm variables"=w361:T14[])
                n113 = Variant To Data(error in=w367, type=FALSE, Variant=w368) -> (data=w360:bool, error out=w366:errorcluster)
                n114 = for {
                  tunnel: w361 -> [w372] mode=indexing
                  tunnel: w360 -> [w371]
                  tunnel: [w370] -> w359 mode=indexing
                  n115 = Bundle By Name(cluster=w372, "Alarm on?"=w371, "Inv 1 over threshold?"=FALSE) -> (w370:T14)
                }
                n116 = Bundle By Name(cluster=w357, "Processing loop variables.ESR alarm variables"=w359) -> (w358:T6)
                n117 = Select(t="Action: Update Alarm & Baseline", s=w360, f="Action: Unset Alarm") -> (s? t:f=w363:string)
              }
              frame "PrivMain.ResetAveraging" {
                n118 = disable-structure shown="Disabled" {
                  disable-tunnel: w377 -> [w380 _]
                  disable-tunnel: w376 -> [w379 w381]
                  disable-tunnel: [w378 w381] -> w375
                  frame Disabled {
                    n119 = Variant To Data(error in=w379, Variant=w380) -> (error out=w378:errorcluster)  [unwired: 1 in, 1 out]
                  }
                  frame Enabled {
                  }
                }
                n120 = local write "reset averaging"(TRUE) -> ()
              }
            }
            n121 = call <vilib>:"Add State(s) to Queue__JKI_lib_State_Machine.vi"("State(s) in Front (\"\")"=w259, "State(s) in (\"\")"=w264) -> ("States Out"=w263:string)  [unwired: 13 in]
          }
        }
      }
      frame "---------- Macro ----------" {
      }
      frame "Macro: Initialize" {
        n122 = call <vilib>:"Add State(s) to Queue__JKI_lib_State_Machine.vi"("State(s) in Front (\"\")"="Initialize\nDE_ Register", "State(s) in (\"\")"=w387) -> ("States Out"=w388:string)  [unwired: 13 in]
      }
      frame "Macro: Exit" {
        n123 = call <vilib>:"Add State(s) to Queue__JKI_lib_State_Machine.vi"("State(s) in Front (\"\")"="DE_Unregister\nAction: FlushDaqQ >> FlushAll\nQuit", "State(s) in (\"\")"=w393) -> ("States Out"=w394:string)  [unwired: 13 in]
      }
      frame "---------- Action ----------" {
        n124 = call <vilib>:"Add State(s) to Queue__JKI_lib_State_Machine.vi"("State(s) in (\"\")"=w398) -> ("States Out"=w399:string)  [unwired: 14 in]
      }
      frame "Action: Update Alarm & Baseline" {
        n125 = disable-structure shown="Enabled" {
          disable-tunnel: [w432 w452] -> w408
          disable-tunnel: w407 -> [w431 w452]
          disable-tunnel: w406 -> [w428 w453]
          disable-tunnel: [w418 w453] -> w405
          disable-tunnel: [w423 _] -> w404
          disable-tunnel: w403 -> [w422 _]
          frame Enabled {
            n126 = Unbundle By Name(w428) -> ("Processing loop variables.Status data"=w421:T36, "Self Reference"=w433:refnum<class "Main.lvclass">)
            n127 = Unbundle By Name(w428) -> ("StoreESR BLine Flag"=w427:bool, "StoredESR Baseline"=w412:dbl[], "UseSavedESR BLine Flag"=w429:bool, "Processing loop variables.DUT INVERTER data"=w416:T37)
            n128 = for {
              tunnel: w416 -> [w435] mode=indexing
              tunnel: [w434] -> w415 mode=indexing
              n129 = Unbundle By Name(w435) -> ("scaled and averaged raw ESR sum"=w434:dbl)
            }
            n130 = call "Get ESR Chart reference.vi"("error in (no error)"=w422, "Main in"=w433) -> ("error out"=w424:errorcluster, "ESR Chart Ref"=w425:refnum<vi>[])  [unwired: 7 in, 1 out]
            n131 = Empty Array?(array=w412) -> (empty?=w413:bool)
            n132 = Select(t=dbl[] [1.0, 1.0, 1.0, 1.0], s=w413, f=w412) -> (s? t:f=w411:dbl[])
            n133 = Select(t=w411, s=w429, f=w415) -> (s? t:f=w414:dbl[])
            n134 = Select(t=w415, s=w427, f=w411) -> (s? t:f=w426:dbl[])
            n135 = Bundle By Name(cluster=w428, "StoredESR Baseline"=w426) -> (w419:T6)
            n136 = Unbundle By Name(w419) -> ("Processing loop variables.ESR alarm variables"=w420:T14[])
            n137 = for {
              tunnel: w425 -> [w444] mode=indexing
              tunnel: w421 -> [w440] mode=indexing
              shift-right: [w441] -> w423
              shift-left: w424 -> [w443]
              tunnel: w420 -> [w439] mode=indexing
              tunnel: [w438] -> w417 mode=indexing
              tunnel: w414 -> [w436] mode=indexing
              n138 = property class="WFChart (strict)"(reference=w444, error in=w443) -> (error out=w441:errorcluster, "YScale.Maximum"=w442:dbl)  [unwired: 1 out]
              n139 = Unbundle By Name(w440) -> ("Inv. 1 on?"=w437:bool)
              n140 = case shown="True" w437 {
                tunnel: w442 -> [_ w451]
                tunnel: w436 -> [w447 w448]
                tunnel: w439 -> [w446 w450]
                tunnel: [w445 w449] -> w438
                frame True {
                  n141 = Bundle By Name(cluster=w446, "Inv 1 baseline ESR"=w447) -> (w445:T14)
                }
                frame False {
                  n142 = Bundle By Name(cluster=w450, "Inv 1 baseline ESR"=w448, "inv 1 esr chart range"=w451) -> (w449:T14)
                }
              }
            }
            n143 = Bundle By Name(cluster=w419, "Processing loop variables.ESR alarm variables"=w417) -> (w418:T6)
            n144 = call <vilib>:"Add State(s) to Queue__JKI_lib_State_Machine.vi"("State(s) in Front (\"\")"="Action: Update ESR Chart Properties\nAction: Reset ESR BLine Flags" ("State(s) in Front (\"\")"), "State(s) in (\"\")"=w431) -> ("States Out"=w432:string)  [unwired: 13 in]
          }
          frame Disabled {
          }
        }
      }
      frame "Action: Update ESR Chart Properties" {
        n145 = Unbundle By Name(w461) -> ("Processing loop variables.DUT INVERTER data"=w460:T37)
        n146 = Unbundle By Name(w461) -> ("StoredESR Baseline"=w456:dbl[], "UseSavedESR BLine Flag"=w467:bool)
        n147 = for {
          tunnel: w460 -> [w473] mode=indexing
          tunnel: [w472] -> w459 mode=indexing
          n148 = Unbundle By Name(w473) -> ("scaled and averaged raw ESR sum"=w472:dbl)
        }
        n149 = Unbundle By Name(w461) -> ("Self Reference"=w468:refnum<class "Main.lvclass">)
        n150 = call "Get ESR Chart reference.vi"("error in (no error)"=w454, "Main in"=w468) -> ("error out"=w465:errorcluster, "ESR Chart Ref"=w466:refnum<vi>[])  [unwired: 7 in, 1 out]
        n151 = Empty Array?(array=w456) -> (empty?=w458:bool)
        n152 = Select(t=dbl[] [1.0, 1.0, 1.0, 1.0], s=w458, f=w456) -> (s? t:f=w455:dbl[])
        n153 = Select(t=w455, s=w467, f=w459) -> (s? t:f=w464:dbl[])
        n154 = Multiply(x=w464, y=4.0) -> (x*y=w462:dbl[])
        n155 = for {
          tunnel: w466 -> [w479] mode=indexing
          tunnel: w462 -> [w477] mode=indexing
          tunnel: w465 -> [w478]
          tunnel: [w480] -> _
          n156 = property class="WFChart (strict)"(reference=w479, error in=w478, "YScale.FormatString"="%.3e", "YScale.Maximum"=w477, "YScale.Minimum"=0.0 ("Y Scale.Range:Minimum"), "History Data"=T35 []) -> (error out=w480:errorcluster)  [unwired: 1 out]
        }
        n157 = call <vilib>:"Add State(s) to Queue__JKI_lib_State_Machine.vi"("State(s) in (\"\")"=w469) -> ("States Out"=w470:string)  [unwired: 14 in]
      }
      frame "Action: Reset ESR BLine Flags" {
        w483 = FALSE ("Value")
        n158 = Unbundle By Name(w486) -> ("Self Reference"=w488:refnum<class "Main.lvclass">)
        n159 = call "Get StoreESR and UseSavedESR Flag reference.vi"("error in (no error)"=w481, "Main in"=w488) -> ("error out"=w485:errorcluster, "UseSavedESR BLine Ref"=w489:refnum<vi>, "StoreESR BLine Ref"=w490:refnum<vi>)  [unwired: 6 in, 1 out]
        n160 = property class="Bool (strict)"(reference=w489, error in=w485, "Value"=w483) -> (error out=w484:errorcluster)  [unwired: 1 out]
        n161 = property class="Bool (strict)"(reference=w490, error in=w484, "Value"=w483) -> (error out=w482:errorcluster)  [unwired: 1 out]
        n162 = Bundle By Name(cluster=w486, "StoreESR BLine Flag"=w483, "UseSavedESR BLine Flag"=w483) -> (w487:T6)
      }
      frame "Action: Unset Alarm" {
        n163 = Unbundle By Name(w498) -> ("Self Reference"=w502:refnum<class "Main.lvclass">)
        n164 = Unbundle By Name(w498) -> ("Processing loop variables.ESR alarm variables"=w496:T14[])
        n165 = call "Get ESR Chart reference.vi"("error in (no error)"=w501, "Main in"=w502) -> ("error out"=w495:errorcluster, "ESR Chart Ref"=w493:refnum<vi>[])  [unwired: 7 in, 1 out]
        n166 = for {
          tunnel: w496 -> [w514] mode=indexing
          tunnel: [w516] -> w500 mode=indexing
          tunnel: FALSE -> [w515]
          tunnel: w496 -> [w513] mode=indexing
          tunnel: w495 -> [w512]
          tunnel: [w508] -> w494
          tunnel: w493 -> [w507] mode=indexing
          n167 = Unbundle By Name(w513) -> ("inv 1 esr chart range"=w506:dbl)
          n168 = Bundle By Name(cluster=w514, "Alarm on?"=w515, "Inv 1 over threshold?"=w515) -> (w516:T14)
          n169 = property class="WFChart (strict)"(reference=w507, error in=w512, "YScale.FormatString"="%#_g", "YScale.Maximum"=w506, "YScale.Minimum"=0.0 ("Y Scale.Range:Minimum"), "History Data"=T35 []) -> (error out=w508:errorcluster)  [unwired: 1 out]
        }
        n170 = call <vilib>:"Add State(s) to Queue__JKI_lib_State_Machine.vi"("State(s) in (\"\")"=w503) -> ("States Out"=w504:string)  [unwired: 14 in]
        n171 = Bundle By Name(cluster=w498, "Processing loop variables.ESR alarm variables"=w500) -> (w497:T6)
      }
      frame "Action: FlushDaqQ" {
        n172 = Unbundle By Name(w518) -> ("RawDaqDataQ"=w520:T10)
        n173 = Flush Queue(queue=w520) -> (error out=w517:errorcluster)  [unwired: 1 in, 2 out]
        n174 = case shown="\"FlushAll\"" w519 {
          tunnel: w518 -> [_ w527]
          tunnel: w517 -> [_ _]
          frame "False", Default {
          }
          frame "FlushAll" {
            n175 = Unbundle By Name(w527) -> ("InverterWaveformsQ"=w524:T11, "InvWfmsQ-DT"=w525:T11, "DPAuxDataQ"=w526:T24)
            n176 = Flush Queue(queue=w526) -> ()  [unwired: 1 in, 3 out]
            n177 = Flush Queue(queue=w525) -> ()  [unwired: 1 in, 3 out]
            n178 = Flush Queue(queue=w524) -> ()  [unwired: 1 in, 3 out]
          }
        }
      }
      frame "Action: ProcessDaqData" {
        n179 = Unbundle By Name(w532) -> ("InvWfmsQ-DT"=w547:T11, "DPAuxDataQ"=w548:T24, "InverterWaveformsQ"=w549:T11)
        n180 = Unbundle By Name(w532) -> ("Acquisition mode"=w530:T20, "Processing loop variables"=w556:T12, "RawDaqDataQ"=w529:T10)
        n181 = Unbundle By Name(w532) -> ("TDMSState"=w551:T23)
        n182 = Unbundle By Name(w532) -> ("LogState"=w533:T22)
        n183 = Not Equal?(x=w551, y=TDMSState--enum."Running") -> (x != y?=w544:bool)
        n184 = Not Equal?(x=w533, y=LogState--enum."Running") -> (x != y?=w531:bool)
        n185 = Get Queue Status(queue=w529, error in (no error)=w538) -> (queue out=w542:T10, error out=w539:errorcluster, # elements in queue=→"RawDaqDataQ size":i32)  [unwired: 1 in, 5 out]
        n186 = Dequeue Element(queue=w542, timeout in ms (-1)=8000, error in (no error)=w539) -> (element=w557:T1, timed out?=w541:bool, error out=w558:errorcluster)  [unwired: 1 out]
        n187 = case shown="False" w541 {
          tunnel: w558 -> [w579 w595]
          tunnel: w557 -> [w574 _]
          tunnel: w556 -> [w576 w594]
          tunnel: "Data Rate 9215 (S/s)" -> [w577 _]
          tunnel: "ESR scaling" -> [w565 _]
          tunnel: "UseDummyVrms" -> [w573 _]
          tunnel: "Dummy Vrms" -> [w572 _]
          tunnel: "reset averaging" -> [w568 _]
          tunnel: w549 -> [w585 _]
          tunnel: w548 -> [w564 _]
          tunnel: w547 -> [w583 _]
          tunnel: [w581 w595] -> w546
          tunnel: "Signal scaling" -> [w575 _]
          tunnel: w544 -> [w570 _]
          tunnel: [w563 w594] -> w536
          tunnel: w531 -> [w569 _]
          tunnel: w530 -> [w567 _]
          tunnel: "Data Rate 9775(S/s)" -> [w566 _]
          frame False {
            w588 = FALSE  # UpdateTS (T)
            n188 = call "Process DAQ Data.vi"("reset averaging"=w568, "Processing loop variables"=w576, "Data Rate 9775(S/s)"=w566, "RawDAQData in"=w574, "Signal scaling"=w575, "error in"=w579, "Data Rate 9215 (S/s)"=w577, "ESR scaling"=w565, "Acquisition mode"=w567, "Use dummy Vout?"=w573, "Dummy Vrms"=w572) -> ("InverterWaveforms"=w571:T38, "Processing loop vars out"=w563:T12, "DataProcAuxData"=w561:T40[], "MeasData"=w562:T41, "error out"=w578:errorcluster)  [unwired: 4 in]
            n189 = case shown="False" w570 {
              tunnel: w585 -> [w592 _]
              tunnel: [w591 errorcluster {"status"=FALSE, "code"=0, "source"=""} ("error constant")] -> w584
              tunnel: w571 -> [w590 _]
              frame False {
                n190 = Enqueue Element(queue=w592, element=w590) -> (error out=w591:errorcluster)  [unwired: 2 in, 2 out]
              }
              frame True {
              }
            }
            n191 = case shown="True" w568 {
              frame False {
              }
              frame True {
                n192 = local write "reset averaging"(FALSE) -> ()
              }
            }
            n193 = call "Set MeasData in Q.vi"("UpdateTS (T)"=w588, "error in (no error)"=w578, "MeasData out"=w562) -> ("error out"=w587:errorcluster)  [unwired: 7 in, 1 out]
            n194 = Enqueue Element(queue=w564, element=w561, error in (no error)=w584) -> (error out=w582:errorcluster)  [unwired: 1 in, 2 out]
            n195 = call "Get MeasData Q and Insert Logging Data.vi"("error in"=w587, "bypass"=w569) -> ("error out"=w586:errorcluster)  [unwired: 6 in, 2 out]
            n196 = Enqueue Element(queue=w583, element=w571, error in (no error)=w582) -> (error out=w580:errorcluster)  [unwired: 1 in, 2 out]
            n197 = Merge Errors(w580, w586) -> (w581:errorcluster)
            "DAQ data" <- w574
          }
          frame True {
          }
        }
        n198 = Bundle By Name(cluster=w532, "Processing loop variables"=w536) -> (w537:T6)
      }
    }
  }
  n199 = while {
    shift-right: [w606] -> _
    shift-left: w3 -> [w605]
    shift-right: [w609] -> w6
    shift-left: w2 -> [w604]
    shift-right: [w608] -> _
    shift-left: w10 -> [w610]
    shift-right: [w603] -> _
    shift-left: _ -> [w602]
    tunnel: w9 -> [w600]
    tunnel: w8 -> [w599]
    tunnel: w4 -> [w598]
    stop <- w607 stop-if-true
    n200 = call <vilib>:"Parse State Queue__JKI_lib_State_Machine.vi"("State Queue"=w610, "Error In (no error)"=w604) -> ("Remaining States"=w612:string, "Current State"=w597:string, "Arguments"=w611:string)  [unwired: 11 in]
    n201 = feedback #2(w598) -> (w596:string)
    n202 = feedback-in #2(w597) -> ()
    n203 = case shown="\"Data: Initialize\"" w597 {
      selector: w597 -> [w614 _ _ _ _ _ _ _ _ _ _ _ _ _ _ _ _ _ _ _ _ _ _ _]
      tunnel: w612 -> [w618 w633 w639 w647 w830 w843 w851 w865 w869 w874 w888 w895 w900 w908 w917 w929 w956 w962 w973 w978 w989 w1019 w1043 w1057]
      tunnel: w611 -> [_ _ _ _ _ _ _ _ _ _ _ _ _ _ w912 w923 _ _ _ _ _ _ w1033 _]
      tunnel: w605 -> [w616 w630 w634 w645 w827 w834 w848 w862 w868 w871 w879 w890 w897 w903 w915 w925 w953 w959 w970 w975 w985 w1015 w1041 w1050]
      tunnel: [w620 errorcluster {"status"=FALSE, "code"=0, "source"=""} ("error out") w637 w644 w828 w840 w844 w863 w866 w872 w886 w891 w898 w904 w913 w926 w954 w960 w971 w976 w980 w1004 w1034 w1045] -> w609
      tunnel: w604 -> [w619 w629 w637 w643 w828 w840 w845 w856 w866 w872 w886 w892 w898 w905 w914 w927 w954 w960 w971 w976 w979 w1003 w1035 w1051]
      tunnel: [w617 w632 w638 w646 w829 w842 w850 w865 w869 w873 w887 w894 w899 w907 w916 w928 w955 w961 w972 w977 w988 w1018 w1042 w1056] -> w608
      tunnel: [_ _ TRUE _ _ _ _ _ _ _ _ _ _ _ _ _ _ _ _ _ _ _ _ _] -> w607
      tunnel: [w616 w630 w634 w642 w827 w841 w848 w862 w868 w871 w882 w890 w897 w903 w915 w925 w953 w959 w970 w975 w985 w1015 w1041 w1050] -> w606
      tunnel: [w613 w627 w635 w640 w826 w831 w849 w864 w867 w870 w881 w889 w896 w906 w911 w922 w952 w958 w964 w974 w987 w1017 w1040 w1055] -> w603
      tunnel: w602 -> [w613 w627 w635 w640 w826 w831 w849 _ w867 w870 w881 w889 w896 w906 w911 w922 w952 w958 w964 w974 w987 w1017 w1040 w1055]
      tunnel: 200 ("Timeout") -> [_ _ _ w641 _ _ _ _ _ _ _ _ _ _ _ _ _ _ _ _ _ _ _ _]
      tunnel: w600 -> [_ _ _ _ _ _ _ _ _ _ _ _ _ _ _ _ _ w957 _ _ _ _ _ _]
      tunnel: w599 -> [_ _ _ _ _ _ _ _ _ _ _ _ _ _ _ _ _ _ w963 _ _ _ _ _]
      tunnel: w596 -> [_ w626 _ _ _ _ _ _ _ _ _ _ _ _ _ _ _ _ _ _ _ _ _ _]
      frame Default {
        w623 = 42 items=["No error", "Argument error", "Memory is full", "Out of zone", "End of file", "File already open", "Generic file I/O error", "File not found", "File permission error", "Disk is full", "Duplicate path", "Too many files open", "System feature not enabled", "Resource file not found", "Cannot add resource", "Resource not found", "Image not found", "Image memory error", "Pen does not exist", "Config type invalid", "Config token not found", "Config parse error", "Config memory error", "Bad external code format", "Bad external code offset", "External code not present", "Null window", "Destroy window error", "Null menu", "Print aborted", "Bad print record", "Print driver error", "Windows error during printing", "Memory error during printing", "Print dialog error", "Generic print error", "Invalid device refnum", "Device not found", "Device parameter error", "Device unit error", "Cannot open device", "Device call aborted", "Generic error", "Cancelled by user", "Object ID too low", "Object ID too high", "Object not in heap", "Unknown heap", "Unknown object (invalid DefProc)", "Unknown object (DefProc not in table)", "Message out of range", "Invalid (null) method", "Unknown message", "Manager call not supported", "Bad address", "Network operation in progress", "Network operation timed out", "Connection is busy", "Network attribute not supported", "Network error", "Address in use", "System out of memory", "Connection aborted", "Connection refused", "Not connected", "Already connected", "Connection closed", "Initialization error (interapplication manager)", "Bad occurrence", "Wait on unbound occurrence handler", "Occurrence queue overflow", "Datalog type conflict", "Unused", "Unrecognized type (interapplication manager)", "Memory corrupt", "Failed to make temporary DLL", "Old CIN version", "Drag socket not found", "Failed to load drop-object", "Failed to register OLE object", "Failed to release OLE object", "Format specifier type mismatch", "Unknown format specifier", "Too few format specifiers", "Too many format specifiers", "Scan failed", "Newer CIN version", "Error converting to variant", "Runtime menu error", "Password tampered", "Variant attribute not found", "Incompatible variant data type", "Event data is not available", "Event Store is not present", "Occurrence is not found", "Event Queue is not created", "Event info is not available", "Refnum passed is NULL", "Error retrieving Class GUID", "Error retrieving CoClass GUID", "Error retrieving TypeLib GUID.", "Bad built application magic bytes.", "Specific driver is different from the specific driver associated with the Logical Name.", "There is no session opened to the class driver.", "Max Error", "MAX - Error with config objects", "MAX - Error loading configuration", "MAX - Group not supported"]
        # "Current State"
        n204 = Format Into String(format string="Software Exception: Unhandled State \"%s\"." ("message"), error in=w619, w614) -> (resulting string=w622:string, error out=w621:errorcluster)  [unwired: 1 in]
        n205 = call <vilib>:"Error Cluster From Error Code.vi"("show call chain? (False)"=TRUE, "error in (no error)"=w621, "error message (\"\")"=w622, "error code (0)"=w623) -> ("error out"=w620:errorcluster)  [unwired: 5 in]
        n206 = call <vilib>:"Add State(s) to Queue__JKI_lib_State_Machine.vi"("State(s) in (\"\")"=w618) -> ("States Out"=w617:string)  [unwired: 14 in]
      }
      frame "Error Handler" {
        n207 = call "General Error Handler - show previous state.vi"("error in (no error)"=w629, "Previous State"=w626, "Loop Select"=enum16{"Event Loop -", "Async Loop -"}."Event Loop -") -> ()  [unwired: 7 in, 2 out]
        n208 = call <vilib>:"Add State(s) to Queue__JKI_lib_State_Machine.vi"("State(s) in Front (\"\")"="/* Post Error States", "State(s) in (\"\")"=w633) -> ("States Out"=w632:string)  [unwired: 13 in]
      }
      frame "Exit" {
        n209 = call <vilib>:"Add State(s) to Queue__JKI_lib_State_Machine.vi"("State(s) in (\"\")"=w639) -> ("States Out"=w638:string)  [unwired: 14 in]
      }
      frame "", "Event Structure", "Idle" {
        n210 = event shown="[5] <Public Events.Main.AsyncCmd Event>: User Event" {
          selector: w640 -> [_ _ _ _ _ _ _ _ _ _ _ _ _]
          dyn-events: _ -> [_ _ _ _ _ _ _ _ _ _ _ _ _]
          timeout: w641 -> [_ _ _ _ _ _ _ _ _ _ _ _ _]
          tunnel: w647 -> [w651 w656 w662 w665 w672 w688 w742 w761 w769 w778 w784 w816 w825]
          tunnel: [w650 w655 w661 w664 w671 w687 w742 w761 w769 w778 w784 w816 w825] -> w646
          tunnel: w645 -> [w648 w653 w659 w667 w675 w677 w733 w756 w764 w772 w783 w811 w820]
          tunnel: [w649 w654 w660 w668 w676 w685 w735 w759 w767 w776 w779 w814 w823] -> w644
          tunnel: w643 -> [w649 w654 w660 w668 w676 w684 w734 w758 w766 w775 w780 w813 w822]
          tunnel: [w648 w653 w659 w667 w674 w679 w736 w757 w765 w774 w783 w812 w821] -> w642
          event Timeout {
            n211 = event-data() -> ()  [unwired: 1 in, 1 out]
            n212 = call <vilib>:"Add State(s) to Queue__JKI_lib_State_Machine.vi"("State(s) in (\"\")"=w651) -> ("States Out"=w650:string)  [unwired: 14 in]
          }
          event "Exit": Value Change {
            n213 = event-data() -> ()  [unwired: 1 in, 1 out]
            n214 = call <vilib>:"Add State(s) to Queue__JKI_lib_State_Machine.vi"("State(s) in Front (\"\")"="Macro: Exit", "State(s) in (\"\")"=w656) -> ("States Out"=w655:string)  [unwired: 13 in]
          }
          event Panel Close? {
            n215 = event-data() -> ()  [unwired: 1 in, 1 out]
            n216 = event-data("Discard?"=TRUE) -> ()  [unwired: 1 in, 1 out]
            n217 = call <vilib>:"Add State(s) to Queue__JKI_lib_State_Machine.vi"("State(s) in Front (\"\")"="Macro: Exit", "State(s) in (\"\")"=w662) -> ("States Out"=w661:string)  [unwired: 13 in]
          }
          event Menu Selection (User) {
            n218 = event-data() -> ("ItemTag"=w666:string)  [unwired: 1 in, 2 out]
            n219 = case shown="\"False\", Default" w666 {
              tunnel: [""] -> w663
              frame "False", Default {
              }
            }
            n220 = call <vilib>:"Add State(s) to Queue__JKI_lib_State_Machine.vi"("State(s) in Front (\"\")"=w663, "State(s) in (\"\")"=w665) -> ("States Out"=w664:string)  [unwired: 13 in]
          }
          event User Event {
            n221 = event-data() -> ("notifier out"=w673:refnum<notifier>)  [unwired: 1 in]
            n222 = Bundle By Name(cluster=w675, "process sync"=w673) -> (w674:T6)
            n223 = call <vilib>:"Add State(s) to Queue__JKI_lib_State_Machine.vi"("State(s) in Front (\"\")"="Macro: Exit", "State(s) in (\"\")"=w672) -> ("States Out"=w671:string)  [unwired: 13 in]
          }
          event User Event {
            n224 = event-data() -> ("CmdMsg"=w682:string, "vData"=w686:variant)  [unwired: 1 in, 1 out]
            n225 = Unbundle By Name(w677) -> ("Self Reference"=w678:refnum<class "Main.lvclass">)
            n226 = call "get async cmd.vi"("error in (no error)"=w684, "Cmd String in"=w682) -> ("error out"=w683:errorcluster, "AsyncCmd"=w681:T47)  [unwired: 8 in]
            n227 = case shown="\"Main.StartProcessing\"" w681 {
              tunnel: w686 -> [_ _ w705 w718]
              tunnel: w683 -> [w694 w696 w699 w726]
              tunnel: [w693 w696 w706 w719] -> w685
              tunnel: [_ _ "Action: StartProcessing" "Action: StopProcessing"] -> w680
              tunnel: w677 -> [w689 w695 w709 w724]
              tunnel: [w689 w695 w708 w723] -> w679
              tunnel: w678 -> [_ _ w701 w722]
              tunnel: w677 -> [_ _ _ _]
              frame Default {
                n228 = call <vilib>:"Build Error Cluster_ModKT .vi"("Prepend String (\"\")"="Invalid Async Cmd" ("Prepend String (\"\")"), "code"=42, "error? (F)"=TRUE, "error in (no error)"=w694) -> ("error out"=w693:errorcluster)  [unwired: 3 in, 1 out]
              }
              frame "Main.RefreshInverterList" {
              }
              frame "Main.StartProcessing" {
                w704 = T48 {"InverterInfo"=[], "ProcessInitParams"=[]}  # StartProcInitParams
                w707 = ProcessingState--enum."Running" ("ProcessingState")
                n229 = disable-structure shown="Enabled" {
                  disable-tunnel: w699 -> [w715 w717]
                  disable-tunnel: [w714 w717] -> _
                  disable-tunnel: w705 -> [w713 _]
                  disable-tunnel: w704 -> [w712 w716]
                  disable-tunnel: [w711 w716] -> w703
                  frame Enabled {
                    n230 = Variant To Data(error in=w715, type=w712, Variant=w713) -> (data=w711:T48, error out=w714:errorcluster)
                  }
                  frame Disabled {
                  }
                }
                n231 = Unbundle(w703) -> ("InverterInfo"=w700:T25[])  [unwired: 1 out]
                n232 = Index Array(array=w700) -> (element=w697:T25)  [unwired: 1 in]
                n233 = property class="Main.lvclass"(reference=w701, error in=w699, "Accessors:InverterInfo*"=w697) -> (reference out=w702:refnum<class "Main.lvclass">, error out=w698:errorcluster)
                n234 = Bundle By Name(cluster=w709, "ProcessingState"=w707, "vData"=w705) -> (w708:T6)
                n235 = call "Fire ProcessingStateChanged Event_DAQ.vi"("error in (no error)"=w698, "DAQState"=w707, "Main in"=w702) -> ("error out"=w706:errorcluster)  [unwired: 7 in, 1 out]
              }
              frame "Main.StopProcessing" {
                w721 = ProcessingState--enum."Idle" ("ProcessingState")
                n236 = disable-structure shown="Enabled" {
                  disable-tunnel: w726 -> [w730 w732]
                  disable-tunnel: [w729 w732] -> w720
                  disable-tunnel: w718 -> [w728 w731]
                  disable-tunnel: [w727 w731] -> _
                  frame Disabled {
                    n237 = Variant To Data(error in=w730, Variant=w728) -> (data=w727:variant, error out=w729:errorcluster)  [unwired: 1 in]
                  }
                  frame Enabled {
                  }
                }
                n238 = call "Fire ProcessingStateChanged Event_DAQ.vi"("error in (no error)"=w720, "DAQState"=w721, "Main in"=w722) -> ("error out"=w719:errorcluster)  [unwired: 7 in, 1 out]
                n239 = Bundle By Name(cluster=w724, "ProcessingState"=w721, "vData"=w718) -> (w723:T6)
              }
            }
            n240 = call <vilib>:"Add State(s) to Queue__JKI_lib_State_Machine.vi"("State(s) in Front (\"\")"=w680, "State(s) in (\"\")"=w688) -> ("States Out"=w687:string)  [unwired: 13 in]
          }
          event User Event {
            n241 = event-data() -> ("CmdMsg"=w741:string, "vData"=w737:variant)  [unwired: 1 in, 1 out]
            n242 = Unbundle By Name(w733) -> ("Self Reference"=w740:refnum<class "Main.lvclass">)
            n243 = call "get async msg.vi"("error in (no error)"=w734, "Msg String in"=w741) -> ("error out"=w738:errorcluster, "AsyncMsg"=w739:T50)  [unwired: 8 in]
            n244 = case shown="\"Main.CurrInverterUpdated\"" w739 {
              tunnel: w740 -> [_ _]
              tunnel: w738 -> [w744 w751]
              tunnel: w737 -> [_ w752]
              tunnel: [w744 w750] -> w735
              tunnel: w733 -> [w743 w749]
              tunnel: [w743 w748] -> w736
              tunnel: w733 -> [_ _]
              frame Default {
              }
              frame "Main.CurrInverterUpdated" {
                w746 = T15 {"name"="", "last updated"=timestamp(0 s since 1904-01-01), "type"="", "inverter Info"={"manufacturer"="", "model"="", "product"="", "serial"="", "power class"="", "year manf"=""}, "gain range"={"gain max"=0.0, "gain min"=0.0, "gain increment"=0.0}, "offset range"={"offset max"=0.0, "offset min"=0.0, "offset increment"=0.0}, "gain actual"=0.0, "offset actual"=0.0, "power level"=0.0, "minimum current"=0.0, "resistance single phase"=0.0, "resistance 3 phase"=0.0, "set flag"=0}  # CurrInverter
                n245 = Build Array(w746) -> (w745:T15[])
                n246 = Variant To Data(error in=w751, type=w745, Variant=w752) -> (data=w747:T15[], error out=w750:errorcluster)
                n247 = Bundle By Name(cluster=w749, "Processing loop variables.CurrInverter"=w747) -> (w748:T6)
              }
            }
          }
          event User Event {
            n248 = event-data() -> ("NEW Settings"=w753:T51)  [unwired: 1 in, 6 out]
            n249 = Unbundle By Name(w756) -> ("Self Reference"=w755:refnum<class "Main.lvclass">)
            n250 = Unbundle By Name(w753) -> ("Measurement config"=w754:T19)
            n251 = call "Fire Private Event.vi"("error in (no error)"=w758, "vData"=w754, "PrivAsync"=PrivateAsynEv_Main--enum."PrivMain.UpdateMeasSettings", "Main in"=w755) -> ("error out"=w759:errorcluster)  [unwired: 6 in, 1 out]
            n252 = Bundle By Name(cluster=w756, "Measurement config"=w754) -> (w757:T6)
          }
          event User Event {
            n253 = event-data() -> ("NEW AcqMode"=w762:T20)  [unwired: 1 in, 6 out]
            n254 = Unbundle By Name(w764) -> ("Self Reference"=w763:refnum<class "Main.lvclass">)
            n255 = call "Fire Private Event.vi"("error in (no error)"=w766, "vData"=w762, "PrivAsync"=PrivateAsynEv_Main--enum."PrivMain.UpdateAcqMode", "Main in"=w763) -> ("error out"=w767:errorcluster)  [unwired: 6 in, 1 out]
            n256 = Bundle By Name(cluster=w764, "Acquisition mode"=w762) -> (w765:T6)
          }
          event User Event {
            n257 = event-data() -> ("NEW State"=w770:T28)  [unwired: 1 in, 6 out]
            n258 = Unbundle By Name(w772) -> ("Self Reference"=w771:refnum<class "Main.lvclass">)
            n259 = Unbundle By Name(w770) -> ("DAQState"=w773:T21)
            n260 = call "Fire Private Event.vi"("error in (no error)"=w775, "vData"=w773, "PrivAsync"=PrivateAsynEv_Main--enum."PrivMain.UpdateDAQState", "Main in"=w771) -> ("error out"=w776:errorcluster)  [unwired: 6 in, 1 out]
            n261 = Bundle By Name(cluster=w772, "DAQState"=w773) -> (w774:T6)
          }
          event User Event {
            n262 = event-data() -> ("ControlLabel"=w782:string, "vData"=w781:variant)  [unwired: 1 in, 1 out]
            n263 = case shown="\"ESR scaling\"" w782 {
              tunnel: w781 -> [_ w791 w796 w801 w807]
              tunnel: w780 -> [w785 w788 w794 w799 w805]
              tunnel: [w785 w787 w793 w798 w804] -> w779
              frame "False", Default {
              }
              frame "ESR scaling" {
                n264 = Build Array(T3 {"Gain"=0.0, "Offset"=0.0} ("ESR scaling")) -> (w786:T3[])
                n265 = Variant To Data(error in=w788, type=w786, Variant=w791) -> (data=w789:T3[], error out=w787:errorcluster)
                n266 = local write "ESR scaling"(w789) -> ()
              }
              frame "UseDummyVrms" {
                n267 = Variant To Data(error in=w794, type=FALSE, Variant=w796) -> (data=w795:bool, error out=w793:errorcluster)
                n268 = local write "UseDummyVrms"(w795) -> ()
              }
              frame "Dummy Vrms" {
                n269 = Variant To Data(error in=w799, type=0.0, Variant=w801) -> (data=w800:dbl, error out=w798:errorcluster)
                n270 = local write "Dummy Vrms"(w800) -> ()
              }
              frame "Signal scaling" {
                n271 = Build Array(T4 {"Iin ripple gain"=13.333, "Iout ripple gain"=13.333, "Iout 60Hz gain "=14.286, "Vout 60Hz gain "=20.0, "Iin ripple offest"=0.0, "Iout ripple offset"=0.0, "Iout 60Hz offset"=0.0, "Vout 60Hz offset"=0.0} ("Signal scaling")) -> (w802:T4[])
                n272 = Variant To Data(error in=w805, type=w802, Variant=w807) -> (data=w806:T4[], error out=w804:errorcluster)
                n273 = local write "Signal scaling"(w806) -> ()
              }
            }
          }
          event User Event {
            n274 = event-data() -> ("NEW State"=w808:T52)  [unwired: 1 in, 6 out]
            n275 = Unbundle By Name(w811) -> ("Self Reference"=w810:refnum<class "Main.lvclass">)
            n276 = Unbundle By Name(w808) -> ("LogState"=w809:T22)
            n277 = call "Fire Private Event.vi"("error in (no error)"=w813, "vData"=w809, "PrivAsync"=PrivateAsynEv_Main--enum."PrivMain.UpdateLogState", "Main in"=w810) -> ("error out"=w814:errorcluster)  [unwired: 6 in, 1 out]
            n278 = Bundle By Name(cluster=w811, "LogState"=w809) -> (w812:T6)
          }
          event User Event {
            n279 = event-data() -> ("NEW State"=w818:T53)  [unwired: 1 in]
            n280 = Unbundle By Name(w820) -> ("Self Reference"=w819:refnum<class "Main.lvclass">)
            n281 = Unbundle By Name(w818) -> ("TDMSState"=w817:T23)
            n282 = call "Fire Private Event.vi"("error in (no error)"=w822, "vData"=w817, "PrivAsync"=PrivateAsynEv_Main--enum."PrivMain.UpdateTDMSState", "Main in"=w819) -> ("error out"=w823:errorcluster)  [unwired: 6 in, 1 out]
            n283 = Bundle By Name(cluster=w820, "TDMSState"=w817) -> (w821:T6)
          }
        }
      }
      frame "---------- Core ----------" {
        n284 = call <vilib>:"Add State(s) to Queue__JKI_lib_State_Machine.vi"("State(s) in (\"\")"=w830) -> ("States Out"=w829:string)  [unwired: 14 in]
      }
      frame "Initialize Core Data" {
        # "originally closed?"
        # "exe?"
        n285 = property class="VI"() -> ("Front Panel.Open"=w839:bool)  [unwired: 2 in, 2 out]
        n286 = property class="App"() -> ("App.Kind"=w838:T43)  [unwired: 2 in, 2 out]
        n287 = control-ref of="Current VI Reference"() -> (w832:refnum<vi>)
        n288 = Not(x=w839) -> (.not. x?=w836:bool)
        n289 = Equal?(x=w838, y=T43."Run Time System" ("Application:Kind")) -> (x = y?=w835:bool)
        n290 = Or(x=w836, y=w835) -> (x .or. y?=w833:bool)
        n291 = Bundle By Name(cluster=w834, "Core.Current VI Reference"=w832, "Core.Close Panel on Exit?"=w833) -> (w841:T6)
        n292 = call <vilib>:"Add State(s) to Queue__JKI_lib_State_Machine.vi"("State(s) in (\"\")"=w843) -> ("States Out"=w842:string)  [unwired: 14 in]
      }
      frame "Process Sync" {
        n293 = Unbundle By Name(w848) -> ("process sync"=w847:refnum<notifier>)
        n294 = Send Notification(notification=TRUE, notifier=w847, error in (no error)=w845) -> (error out=w844:errorcluster)  [unwired: 1 out]
        n295 = call <vilib>:"Add State(s) to Queue__JKI_lib_State_Machine.vi"("State(s) in (\"\")"=w851) -> ("States Out"=w850:string)  [unwired: 14 in]
      }
      frame "DE_Register" {
        n296 = Unbundle By Name(w862) -> ("Public Events"=w861:T9, "PrivateAsync Ev"=w858:refnum<user-event>, "Dependency.DAQ"=w860:refnum<class "DAQ_Engine.lvclass">, "Dependency.Log_Engine"=w857:refnum<class "Log_Engine.lvclass">)
        n297 = property class="DAQ_Engine.lvclass"(reference=w860, error in=w856) -> (error out=w853:errorcluster, "Accessors:PublicEvents*"=w859:T54)  [unwired: 1 out]
        n298 = property class="Log_Engine.lvclass"(reference=w857, error in=w856) -> (error out=w854:errorcluster, "Accessors:PublicEvents*"=w855:T55)  [unwired: 1 out]
        n299 = Merge Errors(w853, w854) -> (w852:errorcluster)
        n300 = register-events(error in=w852, w861, w859, w858, w855) -> (reference out=w864:refnum<event-registration>, error out=w863:errorcluster)  [unwired: 1 in]
      }
      frame "DE_Unregister" {
        n301 = Unregister For Events(event registration refnum=w867, error in=w866) -> ()  [unwired: 1 out]
      }
      frame "---------- Data ----------" {
        n302 = call <vilib>:"Add State(s) to Queue__JKI_lib_State_Machine.vi"("State(s) in (\"\")"=w874) -> ("States Out"=w873:string)  [unwired: 14 in]
      }
      frame "Data: Initialize" {
        w883 = T56 {"Current VI Reference"=refnum, "Close Panel on Exit?"=FALSE}  # Core
        w885 = TRUE  # Your Boolean data
        w884 = ""  # Your string data
        # "#NOTE: possibly get this from Main UI instead."
        n303 = Unbundle By Name(w879) -> ("Settings.Signal scaling"=w880:T4[])
        n304 = Unbundle By Name(w879) -> ("Dependency.DAQ"=w878:refnum<class "DAQ_Engine.lvclass">)
        n305 = property class="DAQ_Engine.lvclass"(reference=w878) -> ("Accessors:MeasSettings*"=w877:T19)  [unwired: 1 in, 2 out]
        n306 = local write "Signal scaling"(w880) -> ()
        n307 = Unbundle By Name(w877) -> ("Data Rate 9215"=w876:dbl, "Data Rate 9775"=w875:dbl)
        n308 = Bundle By Name(cluster=w879, "Core"=w883, "Your Boolean data"=w885, "Your string data"=w884) -> (w882:T6)
        n309 = local write "Data Rate 9215 (S/s)"(w876) -> ()
        n310 = local write "Data Rate 9775(S/s)"(w875) -> ()
        n311 = call <vilib>:"Add State(s) to Queue__JKI_lib_State_Machine.vi"("State(s) in (\"\")"=w888) -> ("States Out"=w887:string)  [unwired: 14 in]
      }
      frame "Data: Cleanup" {
        n312 = Unbundle By Name(w890) -> ("Core.Current VI Reference"=w893:refnum<vi>)
        n313 = Close Reference(reference=w893, error in (no error)=w892) -> (error out=w891:errorcluster)
        n314 = call <vilib>:"Add State(s) to Queue__JKI_lib_State_Machine.vi"("State(s) in (\"\")"=w895) -> ("States Out"=w894:string)  [unwired: 14 in]
      }
      frame "---------- UI ----------" {
        n315 = call <vilib>:"Add State(s) to Queue__JKI_lib_State_Machine.vi"("State(s) in (\"\")"=w900) -> ("States Out"=w899:string)  [unwired: 14 in]
      }
      frame "UI: Initialize" {
        n316 = Unbundle By Name(w903) -> ("Core.Current VI Reference"=w902:refnum<vi>)
        n317 = call <userlib>:"Fit VI window to Largest Dec__ogtk.vi"("error in (no error)"=w905, "VI Ref (calling VI)"=w902) -> ("error out"=w904:errorcluster, "dup VI Ref"=w901:refnum<vi>)  [unwired: 4 in]
        n318 = disable-structure shown="Disabled" {
          disable-tunnel: w901 -> [w910 _]
          frame Disabled {
            n319 = property class="VI"(reference=w910, "Front Panel.Title"="*VI Title*" ("Front Panel Window:Title")) -> ()  [unwired: 1 in, 2 out]
          }
          frame Enabled {
          }
        }
        n320 = call <vilib>:"Add State(s) to Queue__JKI_lib_State_Machine.vi"("State(s) in (\"\")"=w908) -> ("States Out"=w907:string)  [unwired: 14 in]
      }
      frame "UI: Cursor Set" {
        # "Argument"
        n321 = case shown="\"Idle\", Default" w912 {
          tunnel: w914 -> [w919 w921]
          tunnel: [w918 w920] -> w913
          frame "Idle", Default {
            n322 = call <vilib>:"Unset Busy.vi"("error in (no error)"=w919) -> ("error out"=w918:errorcluster)  [unwired: 10 in]
          }
          frame "Busy" {
            n323 = call <vilib>:"Set Busy.vi"("error in (no error)"=w921) -> ("error out"=w920:errorcluster)  [unwired: 9 in, 1 out]
          }
        }
        n324 = call <vilib>:"Add State(s) to Queue__JKI_lib_State_Machine.vi"("State(s) in (\"\")"=w917) -> ("States Out"=w916:string)  [unwired: 14 in]
      }
      frame "UI: Front Panel State" {
        # "Argument"
        n325 = Unbundle By Name(w925) -> ("Core.Current VI Reference"=w924:refnum<vi>)
        n326 = case shown="\"Close\"" w923 {
          tunnel: w927 -> [w933 w946]
          tunnel: [w935 w947] -> w926
          tunnel: w924 -> [w934 w944]
          frame "Open", Default {
            n327 = property class="VI"(reference=w934, error in=w933) -> (reference out=w931:refnum<vi>, error out=w932:errorcluster, "Front Panel.Open"=w930:bool)
            n328 = case shown="False" w930 {
              tunnel: [w938 w941] -> w935
              tunnel: w932 -> [w937 w941]
              tunnel: w931 -> [w936 _]
              frame False {
                n329 = invoke class="VI" method="FP.Open"(reference=w936, error in=w937, "Activate"=TRUE, "State"=T44."Standard") -> (error out=w938:errorcluster)  [unwired: 1 in, 4 out]
              }
              frame True {
              }
            }
          }
          frame "Close" {
            n330 = property class="VI"(reference=w944, error in=w946) -> (reference out=w943:refnum<vi>, error out=w945:errorcluster, "Front Panel.Open"=w942:bool)
            n331 = case shown="True" w942 {
              tunnel: [w948 w951] -> w947
              tunnel: w945 -> [w948 w950]
              tunnel: w943 -> [_ w949]
              frame False {
              }
              frame True {
                n332 = invoke class="VI" method="FP.Close"(reference=w949, error in=w950) -> (error out=w951:errorcluster)  [unwired: 1 in, 2 out]
              }
            }
          }
        }
        n333 = call <vilib>:"Add State(s) to Queue__JKI_lib_State_Machine.vi"("State(s) in (\"\")"=w929) -> ("States Out"=w928:string)  [unwired: 14 in]
      }
      frame "---------- Macro ----------" {
        n334 = call <vilib>:"Add State(s) to Queue__JKI_lib_State_Machine.vi"("State(s) in (\"\")"=w956) -> ("States Out"=w955:string)  [unwired: 14 in]
      }
      frame "Macro: Initialize" {
        n335 = call <vilib>:"Add State(s) to Queue__JKI_lib_State_Machine.vi"("State(s) in Front (\"\")"=w957, "State(s) in (\"\")"=w962) -> ("States Out"=w961:string)  [unwired: 13 in]
      }
      frame "Macro: Exit" {
        n336 = Unbundle By Name(w970) -> ("Core.Close Panel on Exit?"=w969:bool)
        n337 = Select(t="UI: Front Panel State >> Close", s=w969, f="") -> (s? t:f=w966:string)
        n338 = call <vilib>:"Add State(s) to Queue__JKI_lib_State_Machine.vi"("State(s) in (\"\")"=w966, "State(s) at Back (\"\")"=w963) -> ("States Out"=w965:string)  [unwired: 13 in]
        n339 = call <vilib>:"Add State(s) to Queue__JKI_lib_State_Machine.vi"("State(s) in Front (\"\")"=w965, "State(s) in (\"\")"=w973) -> ("States Out"=w972:string)  [unwired: 13 in]
      }
      frame "---------- Action ----------" {
        n340 = call <vilib>:"Add State(s) to Queue__JKI_lib_State_Machine.vi"("State(s) in (\"\")"=w978) -> ("States Out"=w977:string)  [unwired: 14 in]
      }
      frame "Action: StopProcessing" {
        n341 = Unbundle By Name(w985) -> ("Self Reference"=w981:refnum<class "Main.lvclass">, "ProcessingState"=w984:T5)  [unwired: 1 out]
        n342 = Bundle("ProcessingState"=w984, "Variant"=variant) -> (w986:cluster{"ProcessingState":T5, "Variant":variant})  [unwired: 1 in]
        n343 = call "Fire Private Event.vi"("error in (no error)"=w979, "vData"=w986, "PrivAsync"=PrivateAsynEv_Main--enum."PrivMain.UpdateProcessingState", "Main in"=w981) -> ("error out"=w980:errorcluster)  [unwired: 6 in, 1 out]
        n344 = call <vilib>:"Add State(s) to Queue__JKI_lib_State_Machine.vi"("State(s) in (\"\")"=w989) -> ("States Out"=w988:string)  [unwired: 14 in]
      }
      frame "Action: StartProcessing" {
        w1013 = T48 {"InverterInfo"=[], "ProcessInitParams"=[]}  # StartProcInitParams
        w1006 = T12 {"DUT ESR avg"=[], "DUT  PF avg"=[], "DUT  Power avg "=[], "DUT processed data"=[], "ESR alarm variables"=[], "Status data"=[], "CurrInverter"=[], "miscellaneous"=[], "DUT INVERTER data"=[]}  # Processing loop variables
        n345 = Unbundle By Name(w1015) -> ("ProcessingState"=w1002:T5, "Self Reference"=w1012:refnum<class "Main.lvclass">, "vData"=w1014:variant)
        n346 = Variant To Data(error in=w1003, type=w1013, Variant=w1014) -> (data=w994:T48, error out=w1010:errorcluster)
        n347 = Unbundle By Name(w994) -> ("InverterInfo"=w993:T25[], "ProcessInitParams"=w992:T49[])
        n348 = for {
          tunnel: [w1021] -> w1007
          tunnel: [w1028] -> w991
          tunnel: [w1027] -> w997 mode=indexing
          tunnel: [w1029] -> w996 mode=indexing
          tunnel: [w1026] -> w990
          tunnel: [w1024] -> w995 mode=indexing
          tunnel: w993 -> [w1021] mode=indexing
          tunnel: w992 -> [w1022] mode=indexing
          n349 = Unbundle By Name(w1022) -> ("MinCurrThreshold"=w1023:dbl, "ESR alarm threshhold (%)"=w1031:dbl, "NumPF RdsToAvg"=w1026:i32, "# readings to average"=w1028:i32)
          n350 = Unbundle By Name(w1021) -> ("Inverter ID"=w1020:string)
          n351 = Bundle By Name(cluster=T14 {"Inv 1 baseline ESR"=0.0, "Inv 1 over threshold?"=FALSE, "Alarm on?"=FALSE, "inv 1 esr chart range"=0.0, "inv 1 esr saved baseline"=0.0, "ESR alarm threshhold"=0.0} ("ESR alarm variables"), "ESR alarm threshhold"=w1031) -> (w1027:T14)
          n352 = Bundle By Name(cluster=T46 {"Inverter 1 ID"="", "Inverter 2 ID"="", "Packet count"=0, "Calibration"=0.0, "Calibration Gain"=0.0, "Calibration Offset"=0.0, "Calculated Total Power"=0.0, "Seconds"=0.0, "Last Tag Event"=0.0, "Tag Event Time"=0.0} ("miscellaneous"), "Inverter 1 ID"=w1020) -> (w1029:T46)
          n353 = Bundle By Name(cluster=T45 {"Inv. 1 on?"=FALSE, "Inv. 1 ESR over threshhold?"=FALSE, "Minimum current"=0.0} ("Status data"), "Minimum current"=w1023) -> (w1024:T45)
        }
        n354 = property class="Main.lvclass"(reference=w1012, error in=w1010, "Accessors:InverterInfo*"=w1007) -> (reference out=w1011:refnum<class "Main.lvclass">, error out=w1009:errorcluster, "Accessors:CurrInverter*"=w998:T15[])
        n355 = Bundle By Name(cluster=w1006, "CurrInverter"=w998, "miscellaneous"=w996, "Status data"=w995, "ESR alarm variables"=w997) -> (w1005:T12)
        n356 = call "initialize averaging variables.vi"("# of  power factor reads to avg"=w990, "error in (no error)"=w1009, "# of ESR reads to  average"=w991, "Processing loop variables"=w1005) -> ("error out"=w1008:errorcluster, "Processing loop variables out"=w1000:T12)  [unwired: 6 in]
        n357 = To Variant(anything=w1000) -> (Variant=w999:variant)
        n358 = Bundle("ProcessingState"=w1002, "Variant"=w999) -> (w1001:cluster{"ProcessingState":T5, "Variant":variant})  [unwired: 1 in]
        n359 = call "Fire Private Event.vi"("error in (no error)"=w1008, "vData"=w1001, "PrivAsync"=PrivateAsynEv_Main--enum."PrivMain.UpdateProcessingState", "Main in"=w1011) -> ("error out"=w1004:errorcluster)  [unwired: 6 in, 1 out]
        n360 = call <vilib>:"Add State(s) to Queue__JKI_lib_State_Machine.vi"("State(s) in (\"\")"=w1019) -> ("States Out"=w1018:string)  [unwired: 14 in]
      }
      frame "Action: Wait" {
        n361 = Scan From String(format string="%d", input string=w1033, error in=w1035, default 1=u32 0) -> (error out=w1039:errorcluster, output 1=w1038:u32)  [unwired: 1 in, 2 out]
        n362 = call <userlib>:"Wait (ms)__ogtk.vi"("error in (no error)"=w1039, "milliseconds to wait"=w1038) -> ("error out"=w1034:errorcluster)  [unwired: 8 in, 1 out]
        n363 = call <vilib>:"Add State(s) to Queue__JKI_lib_State_Machine.vi"("State(s) in (\"\")"=w1043) -> ("States Out"=w1042:string)  [unwired: 14 in]
      }
      frame "Action: Terminate AsyncLoop" {
        n364 = Unbundle By Name(w1050) -> ("SMQ"=w1054:refnum<queue>)
        n365 = Unbundle By Name(w1050) -> ("Self Reference"=w1049:refnum<class "Main.lvclass">)
        n366 = Flush Queue(queue=w1054) -> (queue out=w1053:refnum<queue>)  [unwired: 1 in, 2 out]
        n367 = call <vilib>:"Add State to Queue with vData.vi"("queue in"=w1053, "state in"="Macro: Exit", "error in"=w1051) -> ("error out"=w1048:errorcluster)  [unwired: 9 in, 3 out]
        n368 = call "Fire Private Event.vi"("error in (no error)"=w1048, "PrivAsync"=PrivateAsynEv_Main--enum."PrivMain.Stop&Terminate", "Main in"=w1049) -> ("error out"=w1047:errorcluster)  [unwired: 7 in, 1 out]
        n369 = call <userlib>:"Wait (ms)__ogtk.vi"("error in (no error)"=w1047, "milliseconds to wait"=u32 1000) -> ("error out"=w1045:errorcluster)  [unwired: 8 in, 1 out]
        n370 = call <vilib>:"Add State(s) to Queue__JKI_lib_State_Machine.vi"("State(s) in (\"\")"=w1057) -> ("States Out"=w1056:string)  [unwired: 14 in]
      }
    }
  }
  n371 = Merge Errors(w6, w5) -> ()  [unwired: 1 out]
